vi "上管柱组件装配.vi"() -> ()   [LabVIEW 2020]
uses:
  Global_Variable/Global.vi
  Database/Global1.vi
  Global_Variable/A131258.vi
  <vilib>/addons/database/Connection.llb/DB Tools Open Connec (String).vi
  <vilib>/addons/database/Connection.llb/Conn Execute.vi
  <vilib>/addons/database/Recordset.llb/Rec Fetch Recordset Data (R).vi
  <vilib>/Utility/config.llb/NI_LVConfig.lvlib
  <vilib>/addons/database/NI_Database_API.lvlib
panel:
  out "USER_ID":string
  out "codeid":string
  out "deviceid":string
  out "productid":string
  out "产品型号":string
  out "联机模式":string
  out "用户权限":string
  out "用户名":string
  in  "轴承压装报表":string[][](table)=[["mm"], ["mm/s"]]
  in  "轴承压装判定结果":bool[][](array[boolean])=[[TRUE]]
  in  "选项卡控件 2":enum32{"轴承压装力位移曲线", "参数查看"}(tab)
  out "判定结果2 2":string
  out "判定结果1 2":string
  out "最小压力下限 2":dbl
  out "最小压力上限 2":dbl
  out "最大压力下限 2":dbl
  out "最大压力上限 2":dbl
  out "位移区间2内最小压力(KN)":dbl
  out "位移区间2内最大压力(KN)":dbl
  out "端铆判定结果45°":string
  out "端铆判定结果0°":string
  out "侧铆判定结果":string
  out "端铆最大压力45°上限":dbl
  out "端铆最大压力0°上限":dbl
  out "侧铆最大压力上限":dbl
  out "端铆最大压力45°下限":dbl
  out "端铆最大压力0°下限":dbl
  out "侧铆最大压力下限":dbl
  in  "质量报警":bool
  in  "设备缺料":bool
  in  "设备故障":bool
  out "端铆最大压力45°(KN)":dbl
  out "端铆最大压力0°(KN)":dbl
  out "侧铆最大压力(KN)":dbl
  out "判定结果3":string
  out "判定结果2":string
  out "判定结果1":string
  out "压装最终位移下限":dbl
  out "压装最终位移上限":dbl
  out "最小压力下限":dbl
  out "最小压力上限":dbl
  out "最大压力下限":dbl
  out "最大压力上限":dbl
  out "压装最终位移(mm)":dbl
  out "不合格指示灯":bool
  out "合格指示灯":bool
  out "位移区间1内最大压力(KN)":dbl
  out "位移区间1内最小压力(KN)":dbl
  out "产品条码":string
  out "轴承压装力位移曲线":cluster{dbl[], dbl[]}[](graph)
  in  "删除":bool
  in  "确定":bool
  in  "添加":bool
  in  "退出":bool
  in  "更新":bool
  in  "产品型号":string(combo)
  in  "选项卡控件 3":enum32{"轴承压装参数", "产品管理", "用户管理"}(tab)
  in  "坐标轴参数":string[][](table)=[["mm"], ["mm/s"]]
  in  "判定框参数":string[][](table)=[["mm"], ["mm/s"]]
  in  "结果判定参数":string[][](table)=[["mm"], ["mm/s"]]
  in  "请输入添加的产品名称":string
  in  "请选择要删除的产品":string(combo)
  in  "进入用户管理":bool
  # "上管柱组件装配"
  # "压装/铆接结果"
  # "下限值"
  # "上限值"
  # "判定结果"
  # "生产结果"
  # "产品二维码"
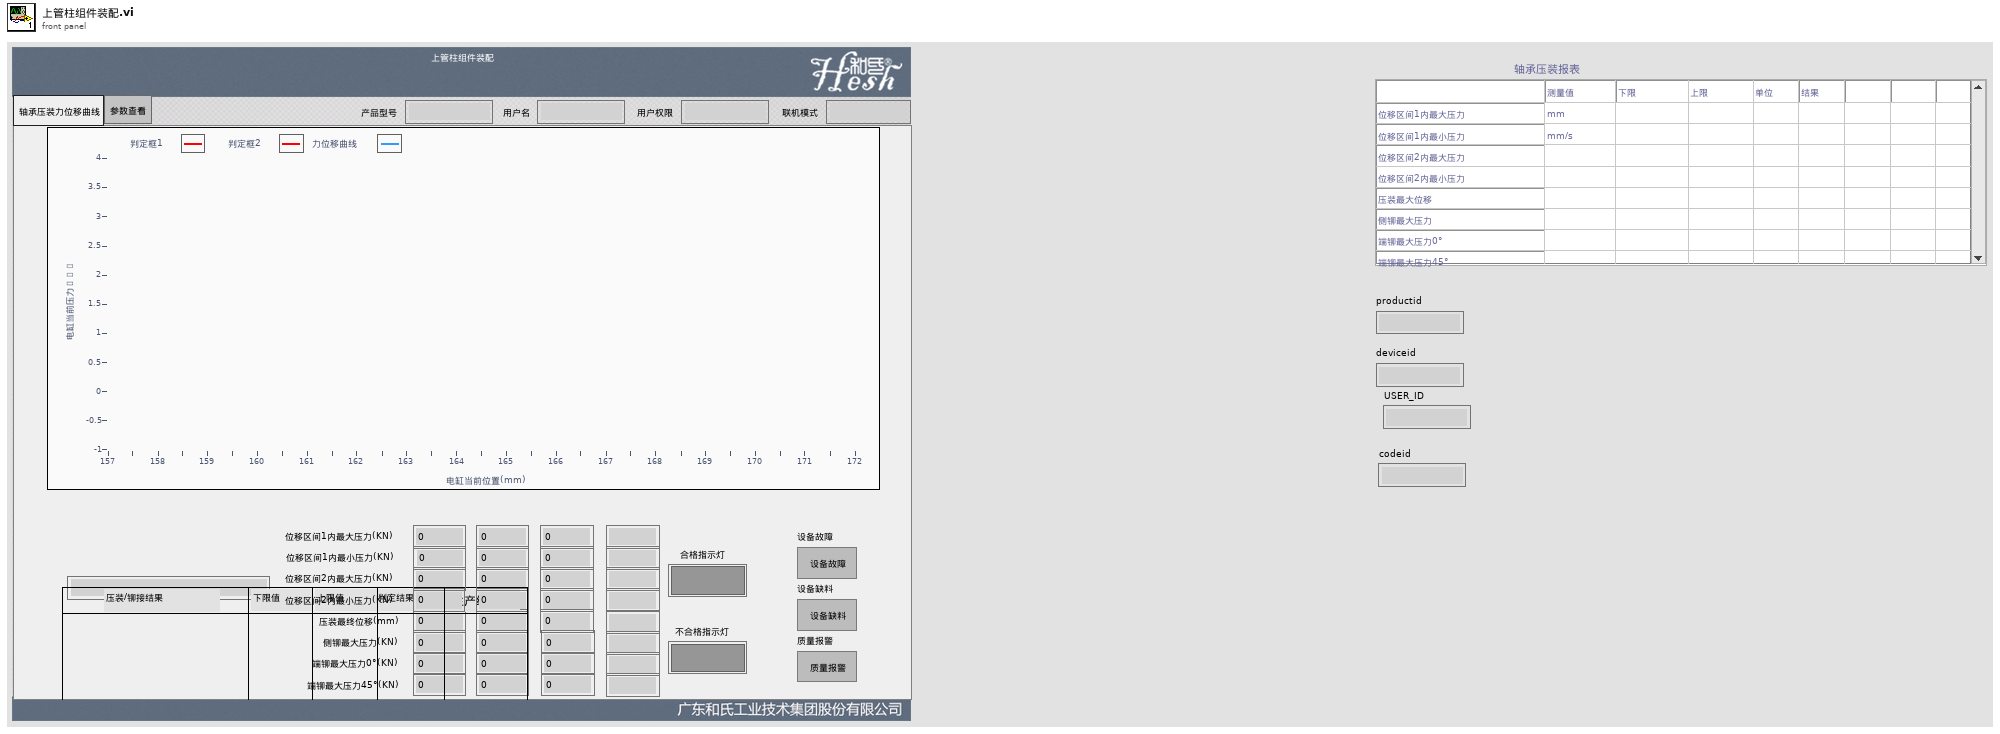
[diagram p1: front panel]
types:
  T1 = enum32{"Invalid", "Standard", "Closed", "Hidden", "Minimized", "Maximized"}
  T2 = cluster{"用户编号":string, "用户名":string, "用户密码(密文)":string, "用户权限":string}
  T3 = cluster{"设备名称":string, "用户名":string, "设备状态":enum16{"设备离线", "设备正常", "设备缺料", "设备故障", "质量报警"}, "附加信息":string}
  T4 = typedef "NI_LVConfig.lvlib/Config Data RefNum.ctl" = refnum<k1>
  T5 = typedef "NI_Database_API.lvlib/Conn ObjectReference.ctl" = refnum<k1>
  T6 = typedef "NI_Database_API.lvlib/Rec ObjectReference.ctl" = refnum<k1>
  T7 = cluster{i64, i64, i64, string, "result string":string}
  T8 = cluster{i64, i64, i64, string, "result string":string}[]
  T9 = cluster{i64, i64, string, "位移区间2内最小压力(KN)":dbl, "最小压力下限 2":dbl, "最小压力上限 2":dbl, string, "判定结果2 2":string}
  T10 = cluster{i64, i64, string, "位移区间2内最大压力(KN)":dbl, "最大压力下限 2":dbl, "最大压力上限 2":dbl, string, "判定结果1 2":string}
  T11 = cluster{i64, i64, string, "压装最终位移(mm) ":dbl, "压装最终位移下限":dbl, "压装最终位移上限":dbl, string, "判定结果3":string}
  T12 = cluster{i64, i64, string, "侧铆最大压力(KN)":dbl, "侧铆最大压力下限":dbl, "侧铆最大压力上限":dbl, string, "侧铆判定结果":string}
  T13 = cluster{i64, i64, string, "位移区间1内最小压力(KN)":dbl, "最小压力下限":dbl, "最小压力上限":dbl, string, "判定结果2":string}
  T14 = cluster{i64, i64, string, "端铆最大压力0°(KN)":dbl, "端铆最大压力0°下限":dbl, "端铆最大压力0°上限":dbl, string, "端铆判定结果0°":string}
  T15 = cluster{i64, i64, string, "位移区间1内最大压力(KN)":dbl, "最大压力下限":dbl, "最大压力上限":dbl, string, "判定结果1":string}
  T16 = cluster{i64, i64, string, "端铆最大压力45°(KN)":dbl, "端铆最大压力45°下限":dbl, "端铆最大压力45°上限":dbl, string, "端铆判定结果45°":string}
  T17 = cluster{i64, i64, string, "端铆最大压力45°(KN)":dbl, "端铆最大压力45°下限":dbl, "端铆最大压力45°上限":dbl, string, "端铆判定结果45°":string}[]
  T18 = cluster{i64, i64, "端铆最大压力45°(KN)":dbl, "端铆最大压力45°下限":dbl, "端铆最大压力45°上限":dbl, string, "端铆判定结果45°":string}
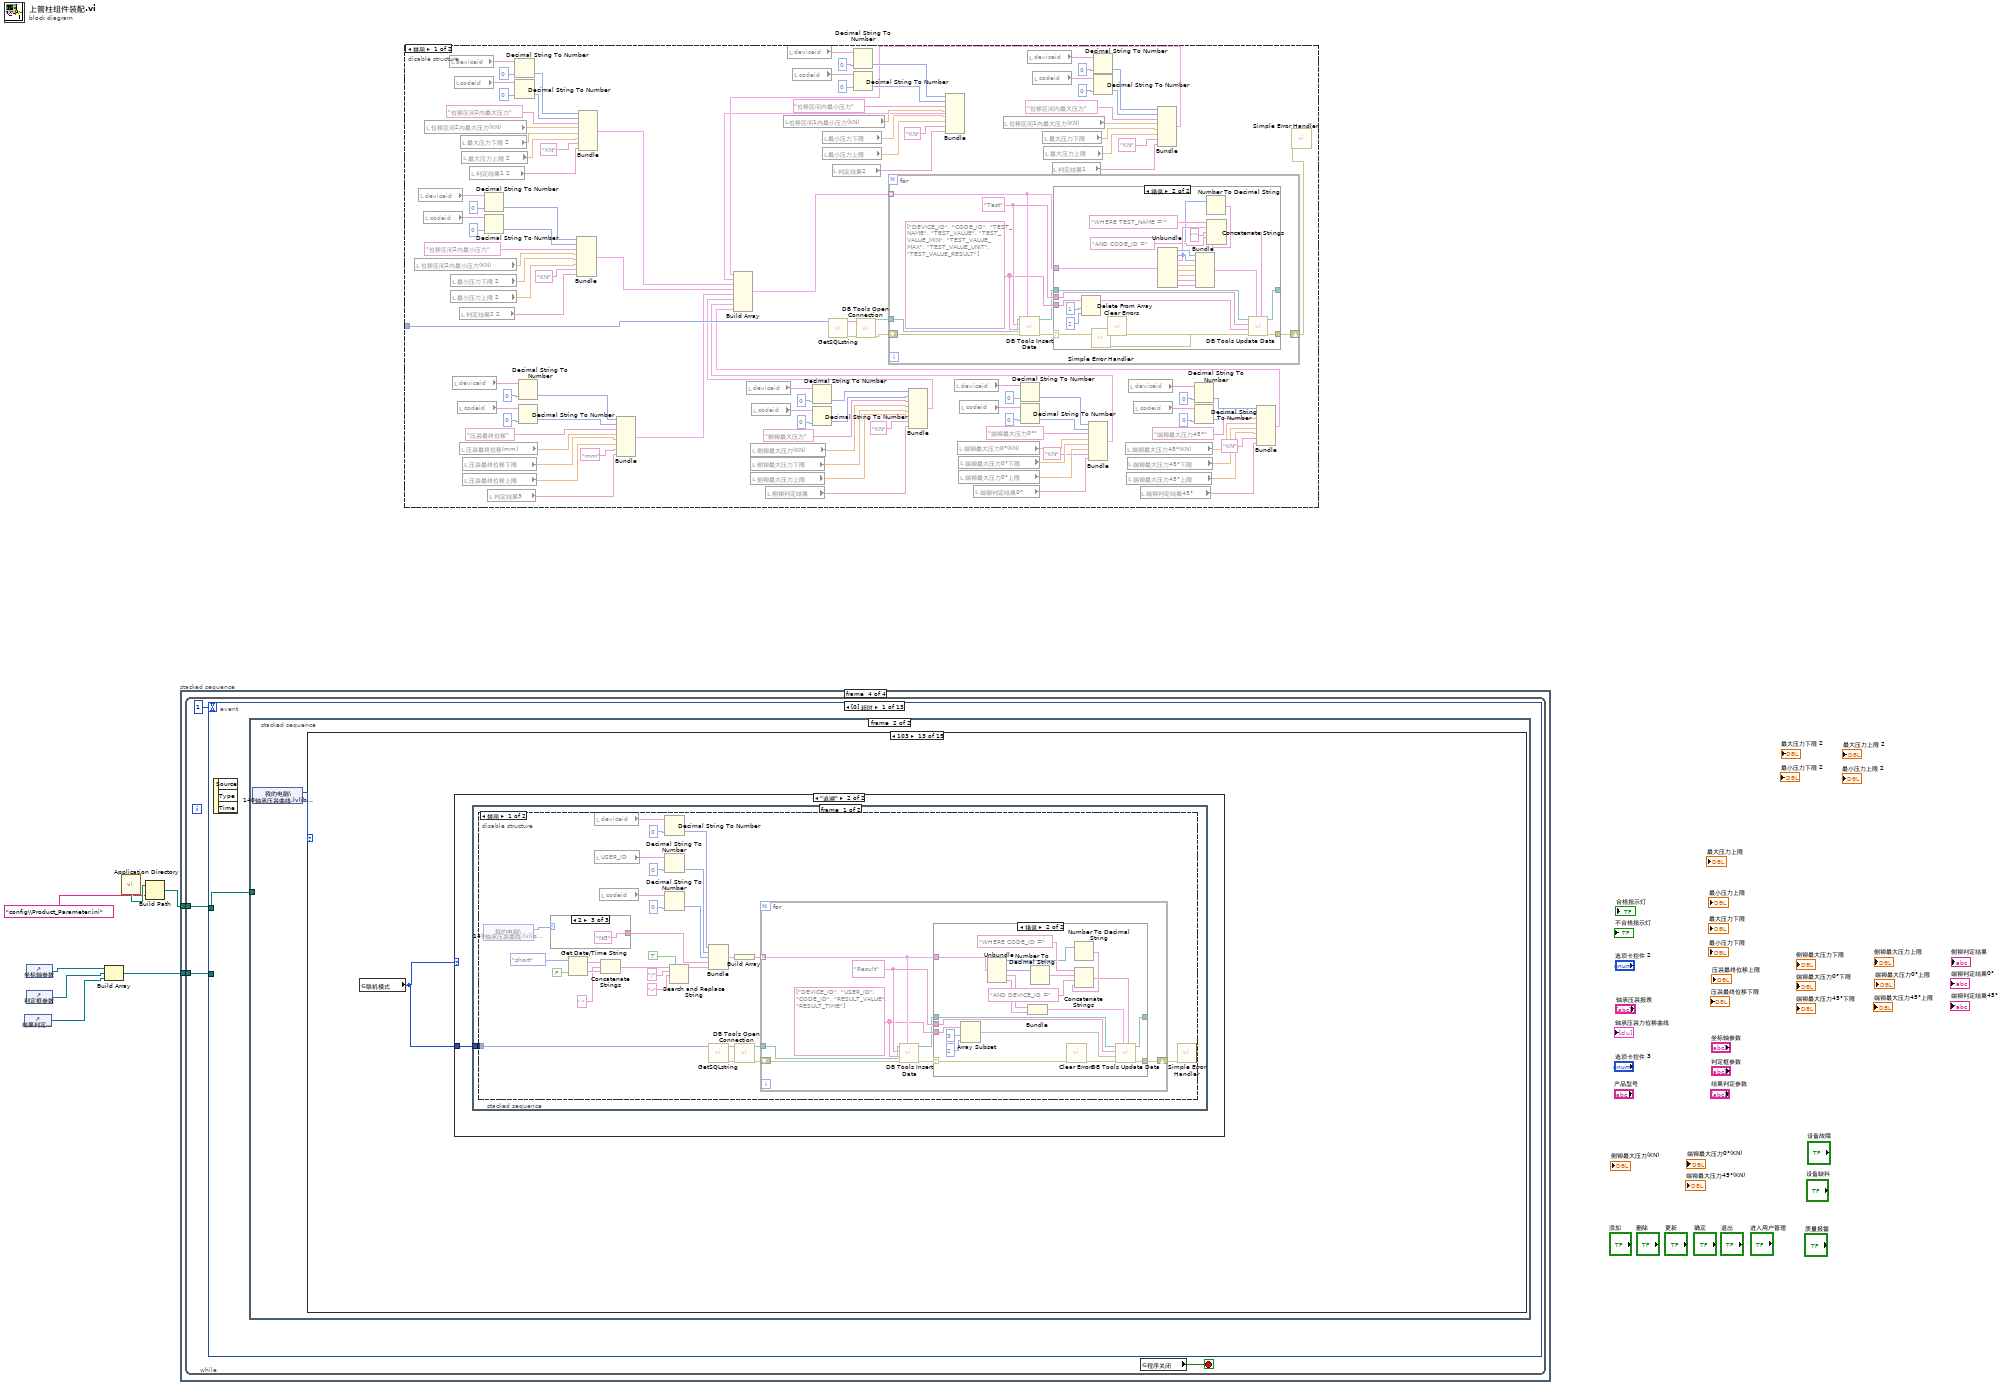
[diagram p0: block diagram]
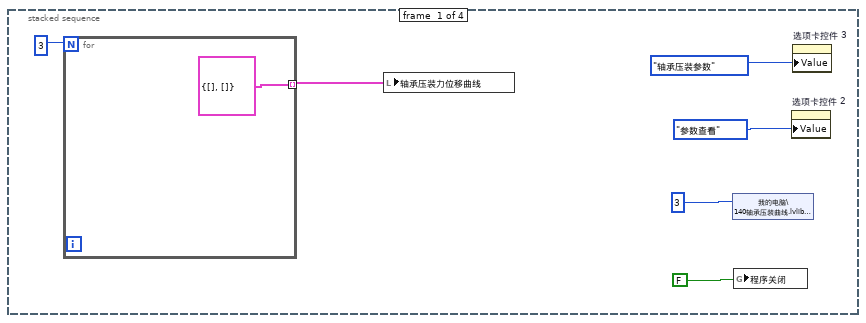
[diagram p4: hidden frame]
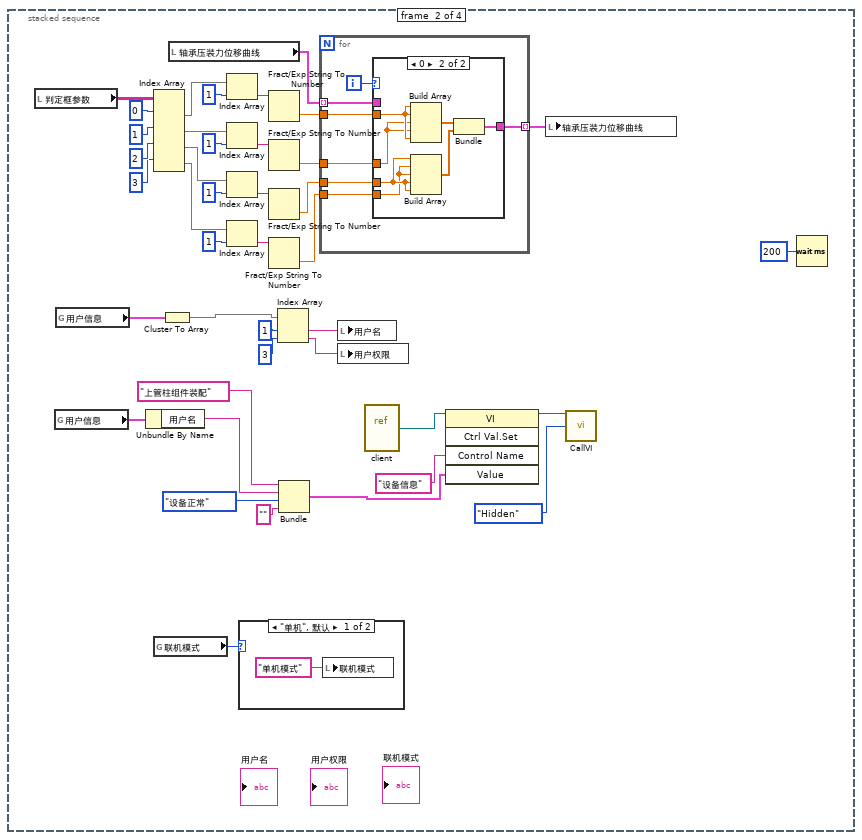
[diagram p5: hidden frame]
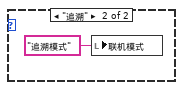
[diagram p6: hidden frame]
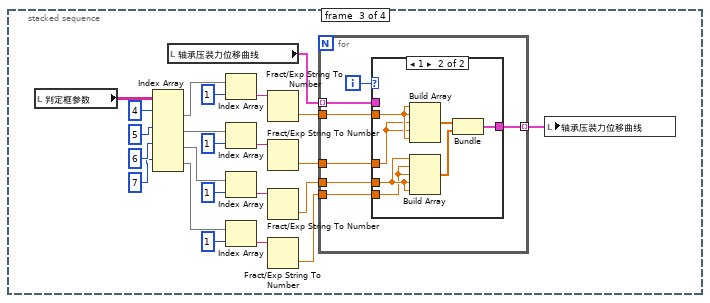
[diagram p8: hidden frame]
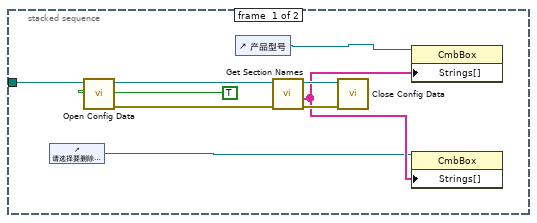
[diagram p10: hidden frame]
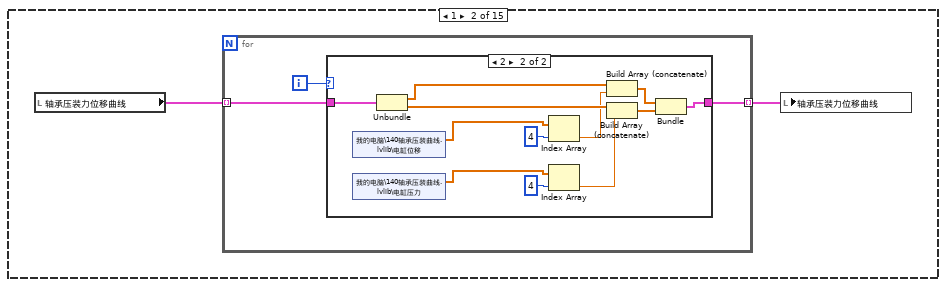
[diagram p12: hidden frame]
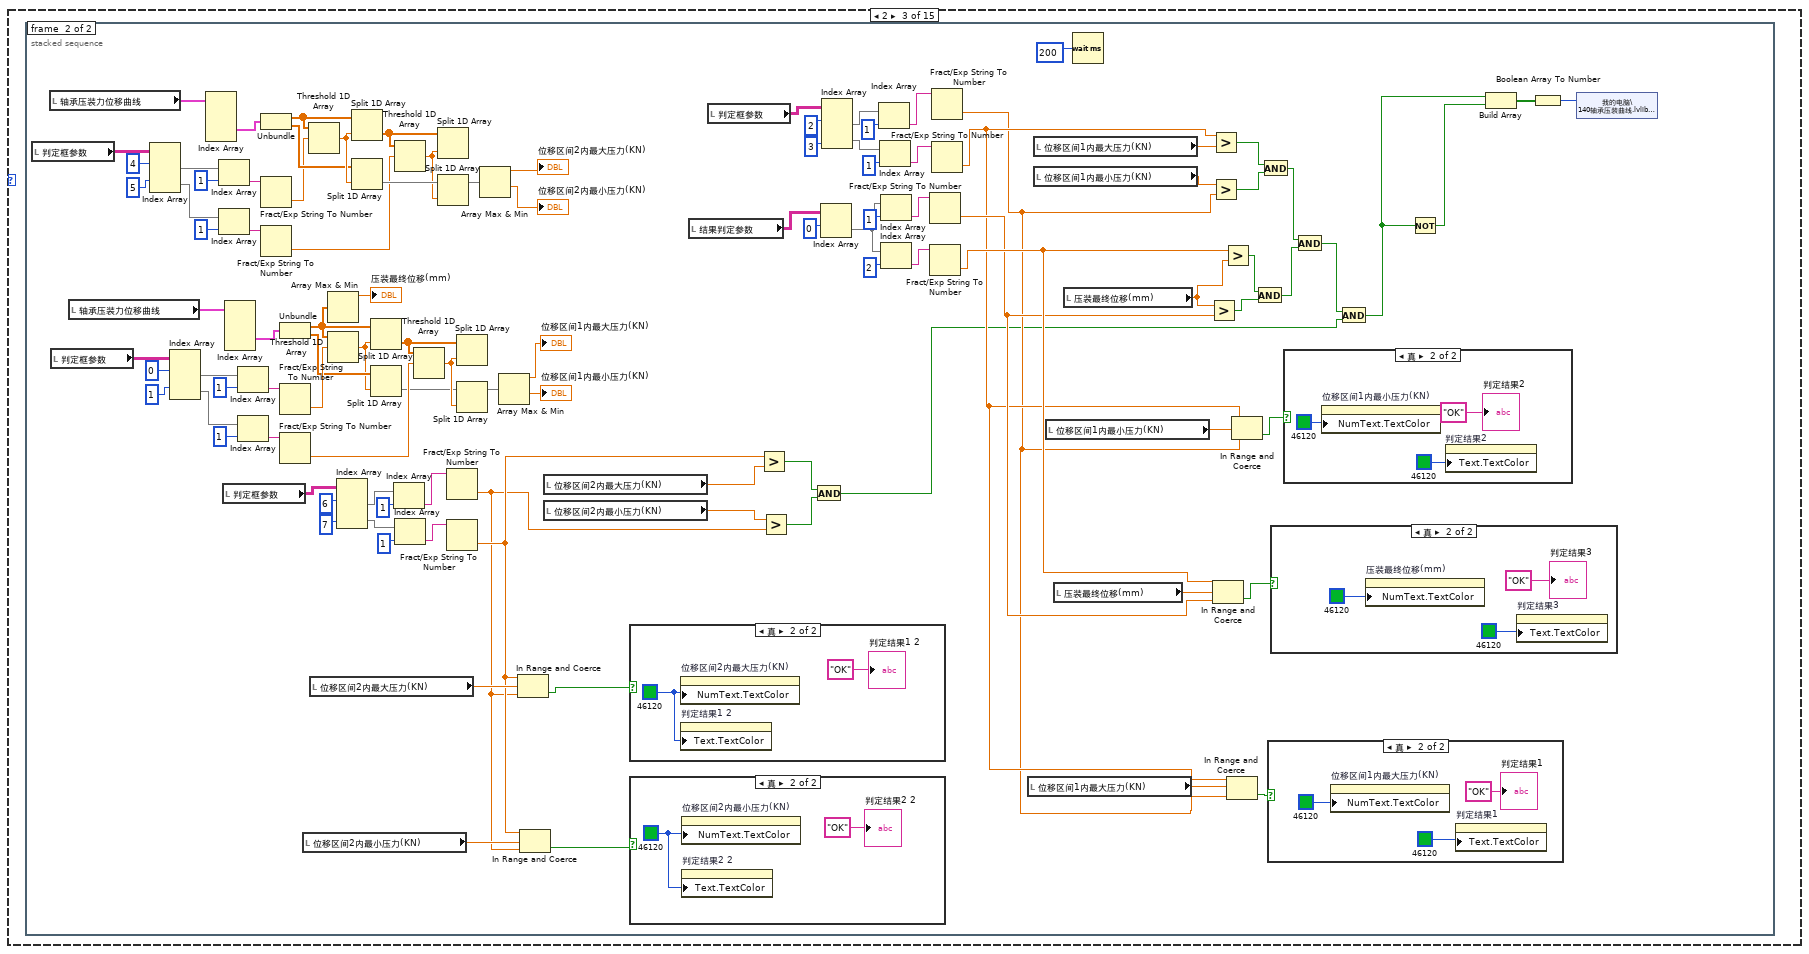
[diagram p14: hidden frame]
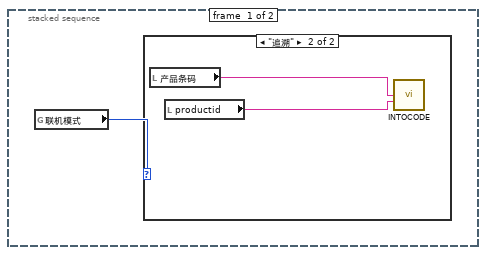
[diagram p15: hidden frame]
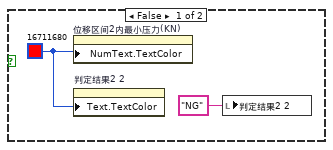
[diagram p17: hidden frame]
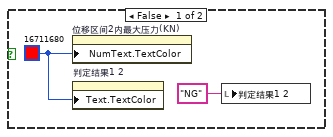
[diagram p18: hidden frame]
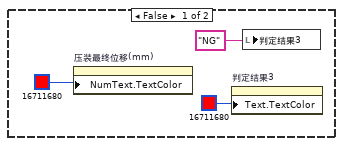
[diagram p19: hidden frame]
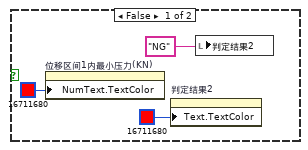
[diagram p20: hidden frame]
diagram:
  n1 = control-ref of="结果判定参数"() -> (w2:refnum<vi>)
  n2 = control-ref of="坐标轴参数"() -> (w4:refnum<vi>)
  n3 = control-ref of="判定框参数"() -> (w3:refnum<vi>)
  n4 = Build Array(w4, w3, w2) -> (w1:refnum<vi>[])
  n5 = call <vilib>:"Application Directory.vi"() -> ("Application Directory"=w7:path)
  n6 = Build Path(base path=w7, name or relative path="config\\Product_Parameter.ini" ("名称或相对路径")) -> (appended path=w5:path)
  n7 = stacked-sequence {
    tunnel: w5 -> [_ _ _ w112]
    tunnel: w1 -> [_ _ _ w111]
    frame #0 {
      n8 = for {
        N: 3 -> [_]
        tunnel: [cluster{dbl[], dbl[]} {[], []}] -> w11 mode=indexing
      }
      n9 = local write "轴承压装力位移曲线"(w11) -> ()
      n10 = shared-variable "我的电脑\\140轴承压装曲线.lvlib\\备用_1"(3) -> ()  [unwired: 1 in, 1 out]
      n11 = global write "Global.vi" "程序关闭"(FALSE ("程序关闭")) -> ()
      n12 = property on="选项卡控件 2" class="TabCtl (严格)"("Value"=enum32{"轴承压装力位移曲线", "参数查看"}."参数查看" ("选项卡控件 2")) -> ()  [unwired: 2 in, 2 out]
      n13 = property on="选项卡控件 3" class="TabCtl (严格)"("Value"=enum32{"轴承压装参数", "产品管理", "用户管理"}."轴承压装参数" ("选项卡控件 3")) -> ()  [unwired: 2 in, 2 out]
    }
    frame #1 {
      n14 = local read "判定框参数"() -> (w53:string[][])
      n15 = global read "Global1.vi" "用户信息"() -> (w23:T2)
      n16 = global read "Global1.vi" "用户信息"() -> (w32:T2)
      n17 = Unbundle By Name(w23) -> ("用户名"=w22:string)
      n18 = Index Array(array=w53, index (row) #1=0 ("索引 (行)"), index (row) #2=1 ("索引 (行)"), index (row) #3=2 ("索引 (行)"), index (row) #4=3 ("索引 (行)")) -> (element #1=w47:string[], element #2=w45:string[], element #3=w43:string[], element #4=w41:string[])  [unwired: 4 in]
      n19 = global read "Global1.vi" "联机模式"() -> (w26:enum16{"单机", "追溯"})
      n20 = Cluster To Array(cluster=w32) -> (array=w31:string[])
      n21 = local read "轴承压装力位移曲线"() -> (w55:cluster{dbl[], dbl[]}[])
      n22 = Index Array(array=w47, index=1 ("索引")) -> (element=w37:string)
      n23 = Index Array(array=w45, index=1 ("索引")) -> (element=w38:string)
      n24 = Index Array(array=w43, index=1 ("索引")) -> (element=w39:string)
      n25 = Index Array(array=w41, index=1 ("索引")) -> (element=w40:string)
      n26 = case shown="\"单机\", 默认" w26 {
        frame "单机", Default {
          n27 = local write "联机模式"("单机模式" ("联机模式")) -> ()
        }
        frame "追溯" {
          n28 = local write "联机模式"("追溯模式" ("联机模式")) -> ()
        }
      }
      n29 = Fract/Exp String To Number(string=w37) -> (number=w36:dbl)  [unwired: 3 in, 1 out]
      n30 = Fract/Exp String To Number(string=w38) -> (number=w35:dbl)  [unwired: 3 in, 1 out]
      n31 = Fract/Exp String To Number(string=w39) -> (number=w34:dbl)  [unwired: 3 in, 1 out]
      n32 = Fract/Exp String To Number(string=w40) -> (number=w33:dbl)  [unwired: 3 in, 1 out]
      n33 = Index Array(array=w31, index #1=1 ("索引"), index #2=3 ("索引")) -> (element #1=w28:string, element #2=w27:string)
      n34 = Bundle("设备名称"="上管柱组件装配", "用户名"=w22, "设备状态"=enum16{"设备离线", "设备正常", "设备缺料", "设备故障", "质量报警"}."设备正常", "附加信息"="") -> (w21:T3)  [unwired: 1 in]
      n35 = for {
        tunnel: [w64] -> w54 mode=indexing
        tunnel: w55 -> [w63] mode=indexing
        tunnel: w36 -> [w61]
        tunnel: w35 -> [w60]
        tunnel: w34 -> [w59]
        tunnel: w33 -> [w58]
        i -> [w62]
        n36 = case shown="0" w62 {
          tunnel: [w65 w70] -> w64
          tunnel: w63 -> [w65 _]
          tunnel: w61 -> [_ w69]
          tunnel: w60 -> [_ w68]
          tunnel: w59 -> [_ w67]
          tunnel: w58 -> [_ w66]
          frame Default {
          }
          frame 0 {
            n37 = Build Array(w69, w69, w68, w68, w69) -> (w71:dbl[])
            n38 = Build Array(w67, w66, w66, w67, w67) -> (w72:dbl[])
            n39 = Bundle(w71, w72) -> (w70:cluster{dbl[], dbl[]})  [unwired: 1 in]
          }
        }
      }
      n40 = local write "用户名"(w28) -> ()
      n41 = local write "用户权限"(w27) -> ()
      n42 = vi-ref "client.vi"() -> (w25:refnum<vi>)
      n43 = invoke class="VI" method="Ctrl Val.Set"(reference=w25, "Control Name"="设备信息" ("控件名"), "Value"=w21) -> (reference out=w24:refnum<vi>)  [unwired: 2 in, 4 out]
      n44 = local write "轴承压装力位移曲线"(w54) -> ()
      n45 = call "CallVI.vi"("VI引用"=w24, "状态"=T1."Hidden") -> ()  [unwired: 11 in, 3 out]
      n46 = Wait (ms)(milliseconds to wait=u32 200 ("等待时间（毫秒）")) -> ()  [unwired: 1 out]
    }
    frame #2 {
      n47 = local read "判定框参数"() -> (w83:string[][])
      n48 = Index Array(array=w83, index (row) #1=4 ("索引 (行)"), index (row) #2=5 ("索引 (行)"), index (row) #3=6 ("索引 (行)"), index (row) #4=7 ("索引 (行)")) -> (element #1=w84:string[], element #2=w85:string[], element #3=w86:string[], element #4=w87:string[])  [unwired: 4 in]
      n49 = local read "轴承压装力位移曲线"() -> (w81:cluster{dbl[], dbl[]}[])
      n50 = Index Array(array=w84, index=1 ("索引")) -> (element=w91:string)
      n51 = Index Array(array=w85, index=1 ("索引")) -> (element=w90:string)
      n52 = Index Array(array=w86, index=1 ("索引")) -> (element=w89:string)
      n53 = Index Array(array=w87, index=1 ("索引")) -> (element=w88:string)
      n54 = Fract/Exp String To Number(string=w91) -> (number=w92:dbl)  [unwired: 3 in, 1 out]
      n55 = Fract/Exp String To Number(string=w90) -> (number=w93:dbl)  [unwired: 3 in, 1 out]
      n56 = Fract/Exp String To Number(string=w89) -> (number=w94:dbl)  [unwired: 3 in, 1 out]
      n57 = Fract/Exp String To Number(string=w88) -> (number=w95:dbl)  [unwired: 3 in, 1 out]
      n58 = for {
        tunnel: [w102] -> w82 mode=indexing
        tunnel: w81 -> [w101] mode=indexing
        tunnel: w92 -> [w99]
        tunnel: w93 -> [w98]
        tunnel: w94 -> [w97]
        tunnel: w95 -> [w96]
        i -> [w100]
        n59 = case shown="1" w100 {
          tunnel: [w103 w108] -> w102
          tunnel: w101 -> [w103 _]
          tunnel: w99 -> [_ w107]
          tunnel: w98 -> [_ w106]
          tunnel: w97 -> [_ w105]
          tunnel: w96 -> [_ w104]
          frame Default {
          }
          frame 1 {
            n60 = Build Array(w107, w107, w106, w106, w107) -> (w109:dbl[])
            n61 = Build Array(w105, w104, w104, w105, w105) -> (w110:dbl[])
            n62 = Bundle(w109, w110) -> (w108:cluster{dbl[], dbl[]})  [unwired: 1 in]
          }
        }
      }
      n63 = local write "轴承压装力位移曲线"(w82) -> ()
    }
    frame #3 {
      n64 = while {
        tunnel: w112 -> [w115]
        tunnel: w111 -> [w116]
        stop <- w113 stop-if-true
        n65 = event shown="[0] 超时" {
          selector: _ -> [_ _ _ _ _ _ _ _ _ _ _ _ _]
          dyn-events: _ -> [_ _ _ _ _ _ _ _ _ _ _ _ _]
          timeout: 1 -> [_ _ _ _ _ _ _ _ _ _ _ _ _]
          tunnel: w115 -> [w117 w769 _ w979 w997 _ w1008 _ _ _ _ _ _]
          tunnel: w116 -> [_ _ _ w978 w996 _ w1007 _ _ _ _ _ _]
          event Timeout {
            n66 = event-data() -> ()  [unwired: 1 in, 3 out]
            n67 = stacked-sequence {
              tunnel: w117 -> [w120 _]
              frame #0 {
                n68 = control-ref of="请选择要删除的产品"() -> (w118:refnum<vi>)
                n69 = call <vilib>:"Open Config Data.vi"("create file if necessary (T)"=TRUE, "configuration file path"=w120) -> ("error out"=w123:errorcluster, "refnum"=w122:T4)  [unwired: 7 in, 1 out]
                n70 = control-ref of="产品型号"() -> (w119:refnum<vi>)
                n71 = call <vilib>:"Get Section Names.vi"("error in (no error)"=w123, "refnum"=w122) -> ("error out"=w125:errorcluster, "section names"=w121:string[], "refnum out"=w124:T4)  [unwired: 7 in]
                n72 = call <vilib>:"Close Config Data.vi"("error in (no error)"=w125, "refnum"=w124) -> ()  [unwired: 8 in, 2 out]
                n73 = property on="属性节点" class="CmbBox"(reference=w119, "Strings[]"=w121) -> ()  [unwired: 1 in, 2 out]
                n74 = property on="属性节点" class="CmbBox"(reference=w118, "Strings[]"=w121) -> ()  [unwired: 1 in, 2 out]
              }
              frame #1 {
                n75 = shared-variable "我的电脑\\140轴承压装曲线.lvlib\\备用_1"() -> (w127:u16)  [unwired: 1 in, 1 out]
                n76 = case shown="103" w127 {
                  frame 0, Default {
                  }
                  frame 1 {
                    n77 = local read "轴承压装力位移曲线"() -> (w128:cluster{dbl[], dbl[]}[])
                    n78 = for {
                      tunnel: [w132] -> w129 mode=indexing
                      tunnel: w128 -> [w131] mode=indexing
                      i -> [w130]
                      n79 = case shown="2" w130 {
                        tunnel: [w133 w139] -> w132
                        tunnel: w131 -> [w133 w138]
                        frame Default {
                        }
                        frame 2 {
                          n80 = shared-variable "我的电脑\\140轴承压装曲线.lvlib\\电缸位移"() -> (w134:sgl[])  [unwired: 1 in, 1 out]
                          n81 = shared-variable "我的电脑\\140轴承压装曲线.lvlib\\电缸压力"() -> (w135:sgl[])  [unwired: 1 in, 1 out]
                          n82 = Unbundle(w138) -> (w143:dbl[], w142:dbl[])
                          n83 = Index Array(array=w134, index=4) -> (element=w136:sgl)
                          n84 = Index Array(array=w135, index=4) -> (element=w137:sgl)
                          n85 = Build Array (concatenate)(w143, w136) -> (w141:dbl[])
                          n86 = Build Array (concatenate)(w142, w137) -> (w140:dbl[])
                          n87 = Bundle(w141, w140) -> (w139:cluster{dbl[], dbl[]})  [unwired: 1 in]
                        }
                      }
                    }
                    n88 = local write "轴承压装力位移曲线"(w129) -> ()
                  }
                  frame 2 {
                    n89 = stacked-sequence {
                      frame #0 {
                        n90 = global read "Global1.vi" "联机模式"() -> (w146:enum16{"单机", "追溯"})
                        n91 = case shown="\"追溯\"" w146 {
                          frame "单机", Default {
                          }
                          frame "追溯" {
                            n92 = local read "产品条码"() -> (w147:string)
                            n93 = local read "productid"() -> (w148:string)
                            n94 = call "INTOCODE.vi"("CODE_MAIN"=w147, "PRODUCT_ID"=w148) -> ()  [unwired: 13 in, 1 out]
                          }
                        }
                      }
                      frame #1 {
                        n95 = local read "判定框参数"() -> (w161:string[][])
                        n96 = local read "轴承压装力位移曲线"() -> (w169:cluster{dbl[], dbl[]}[])
                        n97 = local read "判定框参数"() -> (w187:string[][])
                        n98 = local read "轴承压装力位移曲线"() -> (w176:cluster{dbl[], dbl[]}[])
                        n99 = Index Array(array=w161, index (row) #1=4 ("索引 (行)"), index (row) #2=5 ("索引 (行)")) -> (element #1=w160:string[], element #2=w159:string[])  [unwired: 2 in]
                        n100 = Index Array(array=w187, index (row) #1=0 ("索引 (行)"), index (row) #2=1 ("索引 (行)")) -> (element #1=w188:string[], element #2=w189:string[])  [unwired: 2 in]
                        n101 = Index Array(array=w169) -> (element #3=w150:cluster{dbl[], dbl[]})  [unwired: 4 in, 3 out]
                        n102 = Index Array(array=w160, index=1 ("索引")) -> (element=w158:string)
                        n103 = Index Array(array=w159, index=1 ("索引")) -> (element=w157:string)
                        n104 = local read "判定框参数"() -> (w208:string[][])
                        n105 = Index Array(array=w176) -> (element #3=w149:cluster{dbl[], dbl[]})  [unwired: 4 in, 3 out]
                        n106 = Index Array(array=w188, index=1 ("索引")) -> (element=w190:string)
                        n107 = Index Array(array=w189, index=1 ("索引")) -> (element=w191:string)
                        n108 = Unbundle(w150) -> (w162:dbl[], w163:dbl[])
                        n109 = Fract/Exp String To Number(string=w158) -> (number=w156:dbl)  [unwired: 3 in, 1 out]
                        n110 = Fract/Exp String To Number(string=w157) -> (number=w155:dbl)  [unwired: 3 in, 1 out]
                        n111 = Unbundle(w149) -> (w185:dbl[], w184:dbl[])
                        n112 = Fract/Exp String To Number(string=w190) -> (number=w192:dbl)  [unwired: 3 in, 1 out]
                        n113 = Fract/Exp String To Number(string=w191) -> (number=w193:dbl)  [unwired: 3 in, 1 out]
                        n114 = local read "位移区间2内最小压力(KN)"() -> (w198:dbl)
                        n115 = Threshold 1D Array(2:w156, 3:w162) -> (0:w168:dbl)  [unwired: 1 in]
                        n116 = local read "位移区间2内最大压力(KN)"() -> (w200:dbl)
                        n117 = Array Max & Min(array=w185) -> (max value=→"压装最终位移(mm)":dbl)  [unwired: 3 out]
                        n118 = Threshold 1D Array(2:w192, 3:w185) -> (0:w177:dbl)  [unwired: 1 in]
                        n119 = Index Array(array=w208, index (row) #1=6 ("索引 (行)"), index (row) #2=7 ("索引 (行)")) -> (element #1=w211:string[], element #2=w213:string[])  [unwired: 2 in]
                        n120 = Split 1D Array(array=w162, index=w168) -> (second subarray=w166:dbl[])  [unwired: 1 out]
                        n121 = Split 1D Array(array=w163, index=w168) -> (second subarray=w167:dbl[])  [unwired: 1 out]
                        n122 = Split 1D Array(array=w185, index=w177) -> (second subarray=w179:dbl[])  [unwired: 1 out]
                        n123 = Split 1D Array(array=w184, index=w177) -> (second subarray=w178:dbl[])  [unwired: 1 out]
                        n124 = Index Array(array=w211, index=1 ("索引")) -> (element=w215:string)
                        n125 = Threshold 1D Array(2:w155, 3:w166) -> (0:w165:dbl)  [unwired: 1 in]
                        n126 = Index Array(array=w213, index=1 ("索引")) -> (element=w216:string)
                        n127 = Threshold 1D Array(2:w193, 3:w179) -> (0:w180:dbl)  [unwired: 1 in]
                        n128 = Split 1D Array(array=w166, index=w165) -> ()  [unwired: 2 out]
                        n129 = Split 1D Array(array=w167, index=w165) -> (first subarray=w164:dbl[])  [unwired: 1 out]
                        n130 = Fract/Exp String To Number(string=w215) -> (number=w195:dbl)  [unwired: 3 in, 1 out]
                        n131 = Fract/Exp String To Number(string=w216) -> (number=w196:dbl)  [unwired: 3 in, 1 out]
                        n132 = Split 1D Array(array=w179, index=w180) -> ()  [unwired: 2 out]
                        n133 = Split 1D Array(array=w178, index=w180) -> (first subarray=w181:dbl[])  [unwired: 1 out]
                        n134 = Array Max & Min(array=w164) -> (max value=→"位移区间2内最大压力(KN)":dbl, min value=→"位移区间2内最小压力(KN)":dbl)  [unwired: 2 out]
                        n135 = Array Max & Min(array=w181) -> (max value=→"位移区间1内最大压力(KN)":dbl, min value=→"位移区间1内最小压力(KN)":dbl)  [unwired: 2 out]
                        n136 = In Range and Coerce(upper limit=w196, x=w200, lower limit=w195) -> (In Range?=w199:bool)  [unwired: 1 out]
                        n137 = In Range and Coerce(upper limit=w196, x=w198, lower limit=w195) -> (In Range?=w197:bool)  [unwired: 1 out]
                        n138 = local read "位移区间2内最大压力(KN)"() -> (w207:dbl)
                        n139 = local read "位移区间2内最小压力(KN)"() -> (w206:dbl)
                        n140 = case shown="真" w199 {
                          frame False {
                            w259 = u32 16711680
                            n141 = property on="位移区间2内最大压力(KN)" class="DigNum (严格)"("NumText.TextColor"=w259) -> ()  [unwired: 2 in, 2 out]
                            n142 = property on="判定结果1 2" class="Str"("Text.TextColor"=w259) -> ()  [unwired: 2 in, 2 out]
                            n143 = local write "判定结果1 2"("NG" ("判定结果1")) -> ()
                          }
                          frame True {
                            w261 = u32 46120
                            n144 = property on="位移区间2内最大压力(KN)" class="DigNum (严格)"("NumText.TextColor"=w261) -> ()  [unwired: 2 in, 2 out]
                            n145 = property on="判定结果1 2" class="Str"("Text.TextColor"=w261) -> ()  [unwired: 2 in, 2 out]
                            "判定结果1 2" <- "OK" ("判定结果1")
                          }
                        }
                        n146 = case shown="真" w197 {
                          frame False {
                            w255 = u32 16711680
                            n147 = property on="位移区间2内最小压力(KN)" class="DigNum (严格)"("NumText.TextColor"=w255) -> ()  [unwired: 2 in, 2 out]
                            n148 = property on="判定结果2 2" class="Str"("Text.TextColor"=w255) -> ()  [unwired: 2 in, 2 out]
                            n149 = local write "判定结果2 2"("NG" ("判定结果1")) -> ()
                          }
                          frame True {
                            w257 = u32 46120
                            n150 = property on="位移区间2内最小压力(KN)" class="DigNum (严格)"("NumText.TextColor"=w257) -> ()  [unwired: 2 in, 2 out]
                            n151 = property on="判定结果2 2" class="Str"("Text.TextColor"=w257) -> ()  [unwired: 2 in, 2 out]
                            "判定结果2 2" <- "OK" ("判定结果1")
                          }
                        }
                        n152 = local read "结果判定参数"() -> (w227:string[][])
                        n153 = local read "判定框参数"() -> (w236:string[][])
                        n154 = Greater?(x=w196, y=w207) -> (0:w205:bool)
                        n155 = Greater?(x=w206, y=w195) -> (0:w204:bool)
                        n156 = And(x=w205, y=w204) -> (x .and. y?=w202:bool)
                        n157 = Index Array(array=w227, index (row)=0 ("索引 (行)")) -> (element=w223:string[])  [unwired: 1 in]
                        n158 = Index Array(array=w236, index (row) #1=2 ("索引 (行)"), index (row) #2=3 ("索引 (行)")) -> (element #1=w233:string[], element #2=w231:string[])  [unwired: 2 in]
                        n159 = Index Array(array=w233, index=1 ("索引")) -> (element=w229:string)
                        n160 = Index Array(array=w231, index=1 ("索引")) -> (element=w228:string)
                        n161 = Index Array(array=w223, index=1 ("索引")) -> (element=w224:string)
                        n162 = Index Array(array=w223, index=2 ("索引")) -> (element=w221:string)
                        n163 = Fract/Exp String To Number(string=w224) -> (number=w219:dbl)  [unwired: 3 in, 1 out]
                        n164 = Fract/Exp String To Number(string=w221) -> (number=w220:dbl)  [unwired: 3 in, 1 out]
                        n165 = Fract/Exp String To Number(string=w229) -> (number=w217:dbl)  [unwired: 3 in, 1 out]
                        n166 = Fract/Exp String To Number(string=w228) -> (number=w218:dbl)  [unwired: 3 in, 1 out]
                        n167 = local read "位移区间1内最大压力(KN)"() -> (w242:dbl)
                        n168 = local read "位移区间1内最大压力(KN)"() -> (w251:dbl)
                        n169 = local read "位移区间1内最小压力(KN)"() -> (w250:dbl)
                        n170 = local read "位移区间1内最小压力(KN)"() -> (w240:dbl)
                        n171 = local read "压装最终位移(mm)"() -> (w238:dbl)
                        n172 = local read "压装最终位移(mm)"() -> (w243:dbl)
                        n173 = Wait (ms)(milliseconds to wait=u32 200 ("等待时间（毫秒）")) -> ()  [unwired: 1 out]
                        n174 = Greater?(x=w243, y=w219) -> (0:w247:bool)
                        n175 = Greater?(x=w218, y=w251) -> (0:w249:bool)
                        n176 = Greater?(x=w250, y=w217) -> (0:w248:bool)
                        n177 = In Range and Coerce(upper limit=w220, x=w238, lower limit=w219) -> (In Range?=w237:bool)  [unwired: 1 out]
                        n178 = Greater?(x=w220, y=w243) -> (0:w244:bool)
                        n179 = In Range and Coerce(upper limit=w218, x=w242, lower limit=w217) -> (In Range?=w241:bool)  [unwired: 1 out]
                        n180 = In Range and Coerce(upper limit=w218, x=w240, lower limit=w217) -> (In Range?=w239:bool)  [unwired: 1 out]
                        n181 = And(x=w244, y=w247) -> (x .and. y?=w245:bool)
                        n182 = And(x=w249, y=w248) -> (x .and. y?=w246:bool)
                        n183 = case shown="真" w241 {
                          frame False {
                            n184 = property on="位移区间1内最大压力(KN)" class="DigNum (严格)"("NumText.TextColor"=u32 16711680) -> ()  [unwired: 2 in, 2 out]
                            n185 = property on="判定结果1" class="Str"("Text.TextColor"=u32 16711680) -> ()  [unwired: 2 in, 2 out]
                            n186 = local write "判定结果1"("NG" ("判定结果1")) -> ()
                          }
                          frame True {
                            n187 = property on="位移区间1内最大压力(KN)" class="DigNum (严格)"("NumText.TextColor"=u32 46120) -> ()  [unwired: 2 in, 2 out]
                            n188 = property on="判定结果1" class="Str"("Text.TextColor"=u32 46120) -> ()  [unwired: 2 in, 2 out]
                            "判定结果1" <- "OK" ("判定结果1")
                          }
                        }
                        n189 = case shown="真" w237 {
                          frame False {
                            n190 = property on="压装最终位移(mm)" class="DigNum (严格)"("NumText.TextColor"=u32 16711680) -> ()  [unwired: 2 in, 2 out]
                            n191 = property on="判定结果3" class="Str"("Text.TextColor"=u32 16711680) -> ()  [unwired: 2 in, 2 out]
                            n192 = local write "判定结果3"("NG" ("判定结果1")) -> ()
                          }
                          frame True {
                            n193 = property on="压装最终位移(mm)" class="DigNum (严格)"("NumText.TextColor"=u32 46120) -> ()  [unwired: 2 in, 2 out]
                            n194 = property on="判定结果3" class="Str"("Text.TextColor"=u32 46120) -> ()  [unwired: 2 in, 2 out]
                            "判定结果3" <- "OK" ("判定结果1")
                          }
                        }
                        n195 = case shown="真" w239 {
                          frame False {
                            n196 = property on="位移区间1内最小压力(KN)" class="DigNum (严格)"("NumText.TextColor"=u32 16711680) -> ()  [unwired: 2 in, 2 out]
                            n197 = property on="判定结果2" class="Str"("Text.TextColor"=u32 16711680) -> ()  [unwired: 2 in, 2 out]
                            n198 = local write "判定结果2"("NG" ("判定结果1")) -> ()
                          }
                          frame True {
                            n199 = property on="位移区间1内最小压力(KN)" class="DigNum (严格)"("NumText.TextColor"=u32 46120) -> ()  [unwired: 2 in, 2 out]
                            n200 = property on="判定结果2" class="Str"("Text.TextColor"=u32 46120) -> ()  [unwired: 2 in, 2 out]
                            "判定结果2" <- "OK" ("判定结果1")
                          }
                        }
                        n201 = And(x=w246, y=w245) -> (x .and. y?=w203:bool)
                        n202 = And(x=w203, y=w202) -> (x .and. y?=w201:bool)
                        n203 = Not(x=w201) -> (.not. x?=w252:bool)
                        n204 = Build Array(w201, w252) -> (w254:bool[])
                        n205 = Boolean Array To Number(Boolean array=w254) -> (number=w253:u32)
                        n206 = shared-variable "我的电脑\\140轴承压装曲线.lvlib\\备用_2"(w253) -> ()  [unwired: 1 in, 1 out]
                      }
                    }
                  }
                  frame 3 {
                    w284 = u32 0
                    w282 = "" ("判定结果2")
                    w296 = u16 0 ("备用_2")
                    w349 = FALSE
                    w283 = nan
                    n207 = local read "判定框参数"() -> (w348:string[][])
                    n208 = local read "判定框参数"() -> (w285:string[][])
                    n209 = shared-variable "我的电脑\\140轴承压装曲线.lvlib\\备用_3"(w296) -> ()  [unwired: 1 in, 1 out]
                    n210 = shared-variable "我的电脑\\140轴承压装曲线.lvlib\\备用_4"(w296) -> ()  [unwired: 1 in, 1 out]
                    n211 = shared-variable "我的电脑\\140轴承压装曲线.lvlib\\备用_5"(w296) -> ()  [unwired: 1 in, 1 out]
                    n212 = shared-variable "我的电脑\\140轴承压装曲线.lvlib\\备用_6"(w296) -> ()  [unwired: 1 in, 1 out]
                    n213 = shared-variable "我的电脑\\140轴承压装曲线.lvlib\\备用_7"(w296) -> ()  [unwired: 1 in, 1 out]
                    n214 = Index Array(array=w348, index (row) #1=2 ("索引 (行)"), index (row) #2=3 ("索引 (行)")) -> (element #1=w345:string[], element #2=w343:string[])  [unwired: 2 in]
                    n215 = Index Array(array=w285, index (row) #1=6 ("索引 (行)"), index (row) #2=7 ("索引 (行)")) -> (element #1=w288:string[], element #2=w290:string[])  [unwired: 2 in]
                    n216 = Index Array(array=w345, index=1 ("索引")) -> (element=w341:string)
                    n217 = Index Array(array=w343, index=1 ("索引")) -> (element=w340:string)
                    n218 = Index Array(array=w288, index=1 ("索引")) -> (element=w292:string)
                    n219 = Index Array(array=w290, index=1 ("索引")) -> (element=w293:string)
                    n220 = Fract/Exp String To Number(string=w341) -> (number=w338:dbl)  [unwired: 3 in, 1 out]
                    n221 = Fract/Exp String To Number(string=w340) -> (number=w339:dbl)  [unwired: 3 in, 1 out]
                    n222 = Fract/Exp String To Number(string=w292) -> (number=w295:dbl)  [unwired: 3 in, 1 out]
                    n223 = Fract/Exp String To Number(string=w293) -> (number=w294:dbl)  [unwired: 3 in, 1 out]
                    n224 = local write "最大压力下限"(w338) -> ()
                    n225 = local write "最小压力下限"(w338) -> ()
                    n226 = local write "最大压力上限"(w339) -> ()
                    n227 = local write "最小压力上限"(w339) -> ()
                    n228 = local write "最大压力下限 2"(w295) -> ()
                    n229 = local write "最小压力下限 2"(w295) -> ()
                    n230 = local write "最大压力上限 2"(w294) -> ()
                    n231 = local write "最小压力上限 2"(w294) -> ()
                    n232 = for {
                      N: 3 -> [_]
                      tunnel: [cluster{dbl[], dbl[]} {[], []}] -> w352 mode=indexing
                    }
                    n233 = local read "结果判定参数"() -> (w333:string[][])
                    n234 = Index Array(array=w333, index (row) #1=0 ("索引 (行)"), index (row) #2=0 ("索引 (行)"), index (row) #3=1 ("索引 (行)"), index (row) #4=1 ("索引 (行)"), index (row) #5=2 ("索引 (行)"), index (row) #6=2 ("索引 (行)"), index (row) #7=3 ("索引 (行)"), index (row) #8=3 ("索引 (行)")) -> (element #1=w337:string[], element #2=w336:string[], element #3=w330:string[], element #4=w329:string[], element #5=w328:string[], element #6=w327:string[], element #7=w326:string[], element #8=w325:string[])  [unwired: 8 in]
                    n235 = local write "轴承压装力位移曲线"(w352) -> ()
                    n236 = shared-variable "我的电脑\\140轴承压装曲线.lvlib\\备用_1"(4) -> ()  [unwired: 1 in, 1 out]
                    n237 = Index Array(array=w337, index=1 ("索引")) -> (element=w335:string)
                    n238 = Index Array(array=w336, index=2 ("索引")) -> (element=w334:string)
                    n239 = Index Array(array=w330, index=1 ("索引")) -> (element=w324:string)
                    n240 = Index Array(array=w329, index=2 ("索引")) -> (element=w323:string)
                    n241 = Index Array(array=w328, index=1 ("索引")) -> (element=w322:string)
                    n242 = Index Array(array=w327, index=2 ("索引")) -> (element=w321:string)
                    n243 = Index Array(array=w326, index=1 ("索引")) -> (element=w320:string)
                    n244 = Index Array(array=w325, index=2 ("索引")) -> (element=w319:string)
                    n245 = local write "不合格指示灯"(w349) -> ()
                    n246 = local write "轴承压装判定结果"(bool[][] [] ("轴承压装判定结果")) -> ()
                    n247 = local write "合格指示灯"(w349) -> ()
                    n248 = Fract/Exp String To Number(string=w335) -> (number=w331:dbl)  [unwired: 3 in, 1 out]
                    n249 = Fract/Exp String To Number(string=w334) -> (number=w332:dbl)  [unwired: 3 in, 1 out]
                    n250 = Fract/Exp String To Number(string=w324) -> (number=w318:dbl)  [unwired: 3 in, 1 out]
                    n251 = Fract/Exp String To Number(string=w323) -> (number=w317:dbl)  [unwired: 3 in, 1 out]
                    n252 = Fract/Exp String To Number(string=w322) -> (number=w316:dbl)  [unwired: 3 in, 1 out]
                    n253 = Fract/Exp String To Number(string=w321) -> (number=w315:dbl)  [unwired: 3 in, 1 out]
                    n254 = Fract/Exp String To Number(string=w320) -> (number=w314:dbl)  [unwired: 3 in, 1 out]
                    n255 = Fract/Exp String To Number(string=w319) -> (number=w313:dbl)  [unwired: 3 in, 1 out]
                    n256 = local write "压装最终位移下限"(w331) -> ()
                    n257 = local write "压装最终位移上限"(w332) -> ()
                    n258 = local write "侧铆最大压力下限"(w318) -> ()
                    n259 = local write "侧铆最大压力上限"(w317) -> ()
                    n260 = local write "端铆最大压力0°下限"(w316) -> ()
                    n261 = local write "端铆最大压力0°上限"(w315) -> ()
                    n262 = local write "端铆最大压力45°下限"(w314) -> ()
                    n263 = local write "端铆最大压力45°上限"(w313) -> ()
                    n264 = local write "位移区间1内最大压力(KN)"(w283) -> ()
                    n265 = local write "位移区间1内最小压力(KN)"(w283) -> ()
                    n266 = local write "位移区间2内最大压力(KN)"(w283) -> ()
                    n267 = local write "位移区间2内最小压力(KN)"(w283) -> ()
                    n268 = local write "端铆最大压力45°(KN)"(w283) -> ()
                    n269 = local write "压装最终位移(mm)"(w283) -> ()
                    n270 = local write "侧铆最大压力(KN)"(w283) -> ()
                    n271 = local write "端铆最大压力0°(KN)"(w283) -> ()
                    n272 = property on="位移区间1内最大压力(KN)" class="DigNum (严格)"("NumText.TextColor"=w284) -> ()  [unwired: 2 in, 2 out]
                    n273 = property on="位移区间1内最小压力(KN)" class="DigNum (严格)"("NumText.TextColor"=w284) -> ()  [unwired: 2 in, 2 out]
                    n274 = property on="压装最终位移(mm)" class="DigNum (严格)"("NumText.TextColor"=w284) -> ()  [unwired: 2 in, 2 out]
                    n275 = property on="侧铆最大压力(KN)" class="DigNum (严格)"("NumText.TextColor"=w284) -> ()  [unwired: 2 in, 2 out]
                    n276 = property on="端铆最大压力0°(KN)" class="DigNum (严格)"("NumText.TextColor"=w284) -> ()  [unwired: 2 in, 2 out]
                    n277 = property on="端铆最大压力45°(KN)" class="DigNum (严格)"("NumText.TextColor"=w284) -> ()  [unwired: 2 in, 2 out]
                    n278 = property on="位移区间2内最大压力(KN)" class="DigNum (严格)"("NumText.TextColor"=w284) -> ()  [unwired: 2 in, 2 out]
                    n279 = property on="位移区间2内最小压力(KN)" class="DigNum (严格)"("NumText.TextColor"=w284) -> ()  [unwired: 2 in, 2 out]
                    n280 = local write "判定结果1"(w282) -> ()
                    n281 = local write "判定结果2"(w282) -> ()
                    n282 = local write "判定结果3"(w282) -> ()
                    n283 = local write "侧铆判定结果"(w282) -> ()
                    n284 = local write "端铆判定结果0°"(w282) -> ()
                    n285 = local write "端铆判定结果45°"(w282) -> ()
                    n286 = local write "判定结果1 2"(w282) -> ()
                    n287 = local write "判定结果2 2"(w282) -> ()
                  }
                  frame 4 {
                    n288 = stacked-sequence {
                      frame #0 {
                        n289 = local read "判定框参数"() -> (w358:string[][])
                        n290 = Index Array(array=w358, index (row) #1=0 ("索引 (行)"), index (row) #2=1 ("索引 (行)"), index (row) #3=2 ("索引 (行)"), index (row) #4=3 ("索引 (行)")) -> (element #1=w369:string[], element #2=w367:string[], element #3=w365:string[], element #4=w363:string[])  [unwired: 4 in]
                        n291 = local read "轴承压装力位移曲线"() -> (w375:cluster{dbl[], dbl[]}[])
                        n292 = Index Array(array=w369, index=1 ("索引")) -> (element=w359:string)
                        n293 = Index Array(array=w367, index=1 ("索引")) -> (element=w360:string)
                        n294 = Index Array(array=w365, index=1 ("索引")) -> (element=w361:string)
                        n295 = Index Array(array=w363, index=1 ("索引")) -> (element=w362:string)
                        n296 = Fract/Exp String To Number(string=w359) -> (number=w357:dbl)  [unwired: 3 in, 1 out]
                        n297 = Fract/Exp String To Number(string=w360) -> (number=w356:dbl)  [unwired: 3 in, 1 out]
                        n298 = Fract/Exp String To Number(string=w361) -> (number=w355:dbl)  [unwired: 3 in, 1 out]
                        n299 = Fract/Exp String To Number(string=w362) -> (number=w354:dbl)  [unwired: 3 in, 1 out]
                        n300 = for {
                          tunnel: [w383] -> w376 mode=indexing
                          tunnel: w375 -> [w382] mode=indexing
                          tunnel: w357 -> [w380]
                          tunnel: w356 -> [w379]
                          tunnel: w355 -> [w378]
                          tunnel: w354 -> [w377]
                          i -> [w381]
                          n301 = case shown="0" w381 {
                            tunnel: [w384 w389] -> w383
                            tunnel: w382 -> [w384 _]
                            tunnel: w380 -> [_ w388]
                            tunnel: w379 -> [_ w387]
                            tunnel: w378 -> [_ w386]
                            tunnel: w377 -> [_ w385]
                            frame Default {
                            }
                            frame 0 {
                              n302 = Build Array(w388, w388, w387, w387, w388) -> (w390:dbl[])
                              n303 = Build Array(w386, w385, w385, w386, w386) -> (w391:dbl[])
                              n304 = Bundle(w390, w391) -> (w389:cluster{dbl[], dbl[]})  [unwired: 1 in]
                            }
                          }
                        }
                        n305 = local write "轴承压装力位移曲线"(w376) -> ()
                      }
                      frame #1 {
                        n306 = Wait (ms)(milliseconds to wait=u32 200 ("等待时间（毫秒）")) -> ()  [unwired: 1 out]
                      }
                      frame #2 {
                        n307 = local read "判定框参数"() -> (w405:string[][])
                        n308 = Index Array(array=w405, index (row) #1=4 ("索引 (行)"), index (row) #2=5 ("索引 (行)"), index (row) #3=6 ("索引 (行)"), index (row) #4=7 ("索引 (行)")) -> (element #1=w413:string[], element #2=w412:string[], element #3=w411:string[], element #4=w410:string[])  [unwired: 4 in]
                        n309 = local read "轴承压装力位移曲线"() -> (w414:cluster{dbl[], dbl[]}[])
                        n310 = Index Array(array=w413, index=1 ("索引")) -> (element=w406:string)
                        n311 = Index Array(array=w412, index=1 ("索引")) -> (element=w407:string)
                        n312 = Index Array(array=w411, index=1 ("索引")) -> (element=w408:string)
                        n313 = Index Array(array=w410, index=1 ("索引")) -> (element=w409:string)
                        n314 = Fract/Exp String To Number(string=w406) -> (number=w404:dbl)  [unwired: 3 in, 1 out]
                        n315 = Fract/Exp String To Number(string=w407) -> (number=w403:dbl)  [unwired: 3 in, 1 out]
                        n316 = Fract/Exp String To Number(string=w408) -> (number=w402:dbl)  [unwired: 3 in, 1 out]
                        n317 = Fract/Exp String To Number(string=w409) -> (number=w401:dbl)  [unwired: 3 in, 1 out]
                        n318 = for {
                          tunnel: [w422] -> w415 mode=indexing
                          tunnel: w414 -> [w421] mode=indexing
                          tunnel: w404 -> [w419]
                          tunnel: w403 -> [w418]
                          tunnel: w402 -> [w417]
                          tunnel: w401 -> [w416]
                          i -> [w420]
                          n319 = case shown="1" w420 {
                            tunnel: [w423 w428] -> w422
                            tunnel: w421 -> [w423 _]
                            tunnel: w419 -> [_ w427]
                            tunnel: w418 -> [_ w426]
                            tunnel: w417 -> [_ w425]
                            tunnel: w416 -> [_ w424]
                            frame Default {
                            }
                            frame 1 {
                              n320 = Build Array(w427, w427, w426, w426, w427) -> (w429:dbl[])
                              n321 = Build Array(w425, w424, w424, w425, w425) -> (w430:dbl[])
                              n322 = Bundle(w429, w430) -> (w428:cluster{dbl[], dbl[]})  [unwired: 1 in]
                            }
                          }
                        }
                        n323 = local write "轴承压装力位移曲线"(w415) -> ()
                      }
                    }
                  }
                  frame 5 {
                    w432 = FALSE
                    w434 = u32 0
                    w435 = "" ("侧铆判定结果")
                    w433 = u16 0 ("备用_1")
                    w436 = nan ("侧铆最大压力(KN)")
                    n324 = shared-variable "我的电脑\\140轴承压装曲线.lvlib\\备用_1"(w433) -> ()  [unwired: 1 in, 1 out]
                    n325 = shared-variable "我的电脑\\140轴承压装曲线.lvlib\\备用_3"(w433) -> ()  [unwired: 1 in, 1 out]
                    n326 = shared-variable "我的电脑\\140轴承压装曲线.lvlib\\备用_4"(w433) -> ()  [unwired: 1 in, 1 out]
                    n327 = shared-variable "我的电脑\\140轴承压装曲线.lvlib\\备用_5"(w433) -> ()  [unwired: 1 in, 1 out]
                    n328 = shared-variable "我的电脑\\140轴承压装曲线.lvlib\\备用_6"(w433) -> ()  [unwired: 1 in, 1 out]
                    n329 = shared-variable "我的电脑\\140轴承压装曲线.lvlib\\备用_7"(w433) -> ()  [unwired: 1 in, 1 out]
                    n330 = local write "侧铆最大压力(KN)"(w436) -> ()
                    n331 = local write "端铆最大压力0°(KN)"(w436) -> ()
                    n332 = local write "端铆最大压力45°(KN)"(w436) -> ()
                    n333 = local write "侧铆判定结果"(w435) -> ()
                    n334 = local write "端铆判定结果0°"(w435) -> ()
                    n335 = local write "端铆判定结果45°"(w435) -> ()
                    n336 = local write "轴承压装判定结果"(bool[][] [] ("轴承压装判定结果")) -> ()
                    n337 = property on="侧铆最大压力(KN)" class="DigNum (严格)"("NumText.TextColor"=w434) -> ()  [unwired: 2 in, 2 out]
                    n338 = property on="端铆最大压力45°(KN)" class="DigNum (严格)"("NumText.TextColor"=w434) -> ()  [unwired: 2 in, 2 out]
                    n339 = property on="端铆最大压力0°(KN)" class="DigNum (严格)"("NumText.TextColor"=w434) -> ()  [unwired: 2 in, 2 out]
                    n340 = local write "不合格指示灯"(w432) -> ()
                    n341 = local write "合格指示灯"(w432) -> ()
                  }
                  frame 10 {
                    n342 = stacked-sequence {
                      frame #0 {
                        n343 = shared-variable "我的电脑\\140轴承压装曲线.lvlib\\压力传感器值"() -> (w448:sgl[])  [unwired: 1 in, 1 out]
                        n344 = local read "侧铆最大压力上限"() -> (w440:dbl)
                        n345 = local read "侧铆最大压力下限"() -> (w439:dbl)
                        n346 = Index Array(array=w448, index=0 ("索引")) -> (element=w437:sgl)
                        n347 = Greater?(x=w440, y=w437) -> (0:w446:bool)
                        n348 = Greater?(x=w437, y=w439) -> (0:w445:bool)
                        n349 = In Range and Coerce(upper limit=w440, x=w437, lower limit=w439) -> (In Range?=w438:bool)  [unwired: 1 out]
                        n350 = local write "侧铆最大压力(KN)"(w437) -> ()
                        n351 = And(x=w446, y=w445) -> (x .and. y?=w443:bool)
                        n352 = case shown="真" w438 {
                          frame False {
                            w449 = u32 16711680
                            n353 = property on="侧铆最大压力(KN)" class="DigNum (严格)"("NumText.TextColor"=w449) -> ()  [unwired: 2 in, 2 out]
                            n354 = property on="侧铆判定结果" class="Str"("Text.TextColor"=w449) -> ()  [unwired: 2 in, 2 out]
                            n355 = local write "侧铆判定结果"("NG" ("侧铆判定结果")) -> ()
                          }
                          frame True {
                            w452 = u32 46120
                            n356 = property on="侧铆最大压力(KN)" class="DigNum (严格)"("NumText.TextColor"=w452) -> ()  [unwired: 2 in, 2 out]
                            n357 = property on="侧铆判定结果" class="Str"("Text.TextColor"=w452) -> ()  [unwired: 2 in, 2 out]
                            n358 = local write "侧铆判定结果"("OK" ("侧铆判定结果")) -> ()
                          }
                        }
                        n359 = Not(x=w443) -> (.not. x?=w442:bool)
                        n360 = Build Array(w443, w442) -> (w444:bool[])
                        n361 = Boolean Array To Number(Boolean array=w444) -> (number=w441:u32)
                        n362 = shared-variable "我的电脑\\140轴承压装曲线.lvlib\\备用_4"(w441) -> ()  [unwired: 1 in, 1 out]
                      }
                      frame #1 {
                        n363 = Wait (ms)(milliseconds to wait=u32 800 ("等待时间（毫秒）")) -> ()  [unwired: 1 out]
                      }
                      frame #2 {
                        n364 = shared-variable "我的电脑\\140轴承压装曲线.lvlib\\备用_7"() -> (w454:u16)  [unwired: 1 in, 1 out]
                        n365 = case shown="0, 默认" w454 {
                          frame 0, Default {
                          }
                          frame 1 {
                            n366 = local write "合格指示灯"(TRUE ("合格指示灯")) -> ()
                            n367 = local write "不合格指示灯"(FALSE ("不合格指示灯")) -> ()
                          }
                          frame 2 {
                            n368 = local write "合格指示灯"(FALSE ("合格指示灯")) -> ()
                            n369 = local write "不合格指示灯"(TRUE ("不合格指示灯")) -> ()
                          }
                        }
                      }
                      frame #3 {
                        n370 = shared-variable "我的电脑\\140轴承压装曲线.lvlib\\备用_1"(100) -> ()  [unwired: 1 in, 1 out]
                      }
                    }
                  }
                  frame 20 {
                    n371 = stacked-sequence {
                      frame #0 {
                        n372 = shared-variable "我的电脑\\140轴承压装曲线.lvlib\\压力传感器值"() -> (w471:sgl[])  [unwired: 1 in, 1 out]
                        n373 = local read "端铆最大压力0°下限"() -> (w462:dbl)
                        n374 = local read "端铆最大压力0°上限"() -> (w463:dbl)
                        n375 = Index Array(array=w471, index=1 ("索引")) -> (element=w460:sgl)
                        n376 = local write "端铆最大压力0°(KN)"(w460) -> ()
                        n377 = Greater?(x=w463, y=w460) -> (0:w469:bool)
                        n378 = Greater?(x=w460, y=w462) -> (0:w468:bool)
                        n379 = In Range and Coerce(upper limit=w463, x=w460, lower limit=w462) -> (In Range?=w461:bool)  [unwired: 1 out]
                        n380 = And(x=w469, y=w468) -> (x .and. y?=w466:bool)
                        n381 = case shown="真" w461 {
                          frame False {
                            w472 = u32 16711680
                            n382 = property on="端铆判定结果0°" class="Str"("Text.TextColor"=w472) -> ()  [unwired: 2 in, 2 out]
                            n383 = property on="端铆最大压力0°(KN)" class="DigNum (严格)"("NumText.TextColor"=w472) -> ()  [unwired: 2 in, 2 out]
                            n384 = local write "端铆判定结果0°"("NG" ("侧铆判定结果")) -> ()
                          }
                          frame True {
                            w474 = u32 46120
                            n385 = property on="端铆判定结果0°" class="Str"("Text.TextColor"=w474) -> ()  [unwired: 2 in, 2 out]
                            n386 = property on="端铆最大压力0°(KN)" class="DigNum (严格)"("NumText.TextColor"=w474) -> ()  [unwired: 2 in, 2 out]
                            n387 = local write "端铆判定结果0°"("OK" ("侧铆判定结果")) -> ()
                          }
                        }
                        n388 = Not(x=w466) -> (.not. x?=w465:bool)
                        n389 = Build Array(w466, w465) -> (w467:bool[])
                        n390 = Boolean Array To Number(Boolean array=w467) -> (number=w464:u32)
                        n391 = shared-variable "我的电脑\\140轴承压装曲线.lvlib\\备用_5"(w464) -> ()  [unwired: 1 in, 1 out]
                      }
                      frame #1 {
                        n392 = Wait (ms)(milliseconds to wait=u32 800 ("等待时间（毫秒）")) -> ()  [unwired: 1 out]
                      }
                      frame #2 {
                        n393 = shared-variable "我的电脑\\140轴承压装曲线.lvlib\\备用_7"() -> (w477:u16)  [unwired: 1 in, 1 out]
                        n394 = case shown="2" w477 {
                          frame 0, Default {
                          }
                          frame 1 {
                            n395 = local write "合格指示灯"(TRUE ("合格指示灯")) -> ()
                            n396 = local write "不合格指示灯"(FALSE ("不合格指示灯")) -> ()
                          }
                          frame 2 {
                            n397 = local write "合格指示灯"(FALSE ("合格指示灯")) -> ()
                            n398 = local write "不合格指示灯"(TRUE ("不合格指示灯")) -> ()
                          }
                        }
                      }
                      frame #3 {
                        n399 = shared-variable "我的电脑\\140轴承压装曲线.lvlib\\备用_1"(100) -> ()  [unwired: 1 in, 1 out]
                      }
                    }
                    n400 = stacked-sequence {
                      frame #0 {
                        n401 = shared-variable "我的电脑\\140轴承压装曲线.lvlib\\压力传感器值"() -> (w494:sgl[])  [unwired: 1 in, 1 out]
                        n402 = local read "端铆最大压力0°下限"() -> (w484:dbl)
                        n403 = local read "端铆最大压力0°上限"() -> (w486:dbl)
                        n404 = Index Array(array=w494, index=1 ("索引")) -> (element=w485:sgl)
                        n405 = Greater?(x=w486, y=w485) -> (0:w492:bool)
                        n406 = Greater?(x=w485, y=w484) -> (0:w491:bool)
                        n407 = In Range and Coerce(upper limit=w486, x=w485, lower limit=w484) -> (In Range?=w483:bool)  [unwired: 1 out]
                        n408 = And(x=w492, y=w491) -> (x .and. y?=w489:bool)
                        n409 = case shown="假" w483 {
                          frame False {
                            w495 = u32 16711680
                            n410 = property on="端铆判定结果0°" class="Str"("Text.TextColor"=w495) -> ()  [unwired: 2 in, 2 out]
                            n411 = property on="端铆最大压力0°(KN)" class="DigNum (严格)"("NumText.TextColor"=w495) -> ()  [unwired: 2 in, 2 out]
                            n412 = flat-sequence {
                              tunnel: "NG" ("侧铆判定结果") -> [w497]
                              frame #0 {
                                n413 = local write "端铆判定结果0°"(w497) -> ()
                              }
                            }
                          }
                          frame True {
                            w498 = u32 46120
                            n414 = property on="端铆判定结果0°" class="Str"("Text.TextColor"=w498) -> ()  [unwired: 2 in, 2 out]
                            n415 = property on="端铆最大压力0°(KN)" class="DigNum (严格)"("NumText.TextColor"=w498) -> ()  [unwired: 2 in, 2 out]
                            n416 = local write "端铆判定结果0°"("OK" ("侧铆判定结果")) -> ()
                          }
                        }
                        n417 = Not(x=w489) -> (.not. x?=w488:bool)
                        n418 = Build Array(w489, w488) -> (w490:bool[])
                        n419 = Boolean Array To Number(Boolean array=w490) -> (number=w487:u32)
                        n420 = shared-variable "我的电脑\\140轴承压装曲线.lvlib\\备用_5"(w487) -> ()  [unwired: 1 in, 1 out]
                      }
                      frame #1 {
                        n421 = Wait (ms)(milliseconds to wait=u32 200 ("等待时间（毫秒）")) -> ()  [unwired: 1 out]
                      }
                      frame #2 {
                        n422 = shared-variable "我的电脑\\140轴承压装曲线.lvlib\\备用_2"() -> (w501:u16)  [unwired: 1 in, 1 out]
                        n423 = case shown="1" w501 {
                          frame 0, Default {
                          }
                          frame 1 {
                            n424 = shared-variable "我的电脑\\140轴承压装曲线.lvlib\\备用_5"() -> (w502:u16)  [unwired: 1 in, 1 out]
                            n425 = case shown="2" w502 {
                              frame 0, Default {
                              }
                              frame 1 {
                                n426 = local write "合格指示灯"(TRUE ("合格指示灯")) -> ()
                                n427 = local write "不合格指示灯"(FALSE ("不合格指示灯")) -> ()
                                n428 = shared-variable "我的电脑\\140轴承压装曲线.lvlib\\备用_7"(u16 1 ("备用_5")) -> ()  [unwired: 1 in, 1 out]
                              }
                              frame 2 {
                                n429 = local write "合格指示灯"(FALSE ("合格指示灯")) -> ()
                                n430 = local write "不合格指示灯"(TRUE ("不合格指示灯")) -> ()
                                n431 = shared-variable "我的电脑\\140轴承压装曲线.lvlib\\备用_7"(u16 2 ("备用_5")) -> ()  [unwired: 1 in, 1 out]
                              }
                            }
                          }
                          frame 2 {
                            n432 = shared-variable "我的电脑\\140轴承压装曲线.lvlib\\备用_4"() -> (w509:u16)  [unwired: 1 in, 1 out]
                            n433 = case shown="1" w509 {
                              frame 0, Default {
                              }
                              frame 1 {
                                n434 = shared-variable "我的电脑\\140轴承压装曲线.lvlib\\备用_7"(u16 2 ("备用_5")) -> ()  [unwired: 1 in, 1 out]
                                n435 = local write "合格指示灯"(FALSE ("合格指示灯")) -> ()
                                n436 = local write "不合格指示灯"(TRUE ("不合格指示灯")) -> ()
                              }
                              frame 2 {
                                n437 = shared-variable "我的电脑\\140轴承压装曲线.lvlib\\备用_7"(u16 2 ("备用_5")) -> ()  [unwired: 1 in, 1 out]
                                n438 = local write "合格指示灯"(FALSE ("合格指示灯")) -> ()
                                n439 = local write "不合格指示灯"(TRUE ("不合格指示灯")) -> ()
                              }
                            }
                          }
                        }
                      }
                    }
                  }
                  frame 30 {
                    n440 = stacked-sequence {
                      frame #0 {
                        n441 = shared-variable "我的电脑\\140轴承压装曲线.lvlib\\压力传感器值"() -> (w537:sgl[])  [unwired: 1 in, 1 out]
                        n442 = shared-variable "我的电脑\\140轴承压装曲线.lvlib\\压力传感器值"() -> (w529:sgl[])  [unwired: 1 in, 1 out]
                        n443 = local read "端铆最大压力45°上限"() -> (w520:dbl)
                        n444 = local read "端铆最大压力45°下限"() -> (w519:dbl)
                        n445 = local read "端铆最大压力0°下限"() -> (w521:dbl)
                        n446 = local read "端铆最大压力0°上限"() -> (w522:dbl)
                        n447 = Index Array(array=w537, index=1 ("索引")) -> (element=w517:sgl)
                        n448 = Index Array(array=w529, index=2 ("索引")) -> (element=w516:sgl)
                        n449 = local write "端铆最大压力0°(KN)"(w517) -> ()
                        n450 = local write "端铆最大压力45°(KN)"(w516) -> ()
                        n451 = Greater?(x=w520, y=w516) -> (0:w527:bool)
                        n452 = Greater?(x=w516, y=w519) -> (0:w526:bool)
                        n453 = Greater?(x=w522, y=w517) -> (0:w535:bool)
                        n454 = Greater?(x=w517, y=w521) -> (0:w534:bool)
                        n455 = And(x=w527, y=w526) -> (x .and. y?=w524:bool)
                        n456 = And(x=w535, y=w534) -> (x .and. y?=w525:bool)
                        n457 = In Range and Coerce(upper limit=w522, x=w517, lower limit=w521) -> (In Range?=w530:bool)  [unwired: 1 out]
                        n458 = In Range and Coerce(upper limit=w520, x=w516, lower limit=w519) -> (In Range?=w518:bool)  [unwired: 1 out]
                        n459 = And(x=w525, y=w524) -> (x .and. y?=w523:bool)
                        n460 = case shown="假" w518 {
                          frame False {
                            w538 = u32 16711680
                            n461 = property on="端铆最大压力45°(KN)" class="DigNum (严格)"("NumText.TextColor"=w538) -> ()  [unwired: 2 in, 2 out]
                            n462 = property on="端铆判定结果45°" class="Str"("Text.TextColor"=w538) -> ()  [unwired: 2 in, 2 out]
                            n463 = local write "端铆判定结果45°"("NG" ("端铆判定结果45°")) -> ()
                          }
                          frame True {
                            w540 = u32 46120
                            n464 = property on="端铆最大压力45°(KN)" class="DigNum (严格)"("NumText.TextColor"=w540) -> ()  [unwired: 2 in, 2 out]
                            n465 = property on="端铆判定结果45°" class="Str"("Text.TextColor"=w540) -> ()  [unwired: 2 in, 2 out]
                            n466 = local write "端铆判定结果45°"("OK" ("端铆判定结果45°")) -> ()
                          }
                        }
                        n467 = case shown="假" w530 {
                          frame False {
                            w542 = u32 16711680
                            n468 = property on="端铆判定结果0°" class="Str"("Text.TextColor"=w542) -> ()  [unwired: 2 in, 2 out]
                            n469 = property on="端铆最大压力0°(KN)" class="DigNum (严格)"("NumText.TextColor"=w542) -> ()  [unwired: 2 in, 2 out]
                            n470 = local write "端铆判定结果0°"("NG" ("侧铆判定结果")) -> ()
                          }
                          frame True {
                            w544 = u32 46120
                            n471 = property on="端铆判定结果0°" class="Str"("Text.TextColor"=w544) -> ()  [unwired: 2 in, 2 out]
                            n472 = property on="端铆最大压力0°(KN)" class="DigNum (严格)"("NumText.TextColor"=w544) -> ()  [unwired: 2 in, 2 out]
                            n473 = local write "端铆判定结果0°"("OK" ("侧铆判定结果")) -> ()
                          }
                        }
                        n474 = Not(x=w523) -> (.not. x?=w532:bool)
                        n475 = Build Array(w523, w532) -> (w533:bool[])
                        n476 = Boolean Array To Number(Boolean array=w533) -> (number=w531:u32)
                        n477 = shared-variable "我的电脑\\140轴承压装曲线.lvlib\\备用_6"(w531) -> ()  [unwired: 1 in, 1 out]
                      }
                      frame #1 {
                        n478 = Wait (ms)(milliseconds to wait=u32 800 ("等待时间（毫秒）")) -> ()  [unwired: 1 out]
                      }
                      frame #2 {
                        n479 = shared-variable "我的电脑\\140轴承压装曲线.lvlib\\备用_7"() -> (w547:u16)  [unwired: 1 in, 1 out]
                        n480 = case shown="2" w547 {
                          frame 0, Default {
                          }
                          frame 1 {
                            n481 = local write "合格指示灯"(TRUE ("合格指示灯")) -> ()
                            n482 = local write "不合格指示灯"(FALSE ("不合格指示灯")) -> ()
                          }
                          frame 2 {
                            n483 = local write "合格指示灯"(FALSE ("合格指示灯")) -> ()
                            n484 = local write "不合格指示灯"(TRUE ("不合格指示灯")) -> ()
                          }
                        }
                      }
                      frame #3 {
                        n485 = shared-variable "我的电脑\\140轴承压装曲线.lvlib\\备用_1"(100) -> ()  [unwired: 1 in, 1 out]
                      }
                    }
                  }
                  frame 100 {
                    n486 = stacked-sequence {
                      frame #0 {
                        w554 = "KN" ("元素")
                        w561 = "KN" ("元素")
                        n487 = local read "位移区间1内最大压力(KN)"() -> (w601:dbl)
                        n488 = local read "位移区间2内最小压力(KN)"() -> (w571:dbl)
                        n489 = local read "最大压力上限"() -> (w603:dbl)
                        n490 = local read "最大压力下限"() -> (w602:dbl)
                        n491 = local read "位移区间2内最大压力(KN)"() -> (w577:dbl)
                        n492 = local read "最小压力下限 2"() -> (w570:dbl)
                        n493 = local read "最小压力上限 2"() -> (w569:dbl)
                        n494 = local read "判定结果2 2"() -> (w559:string)
                        n495 = local read "判定结果1"() -> (w563:string)
                        n496 = local read "最大压力上限 2"() -> (w575:dbl)
                        n497 = local read "最大压力下限 2"() -> (w576:dbl)
                        n498 = Number To Fractional String(number=w601) -> (F-format string=w610:string)  [unwired: 3 in]
                        n499 = Number To Fractional String(number=w602) -> (F-format string=w611:string)  [unwired: 3 in]
                        n500 = Number To Fractional String(number=w603) -> (F-format string=w612:string)  [unwired: 3 in]
                        n501 = Number To Fractional String(number=w571) -> (F-format string=w568:string)  [unwired: 3 in]
                        n502 = Number To Fractional String(number=w570) -> (F-format string=w567:string)  [unwired: 3 in]
                        n503 = Number To Fractional String(number=w569) -> (F-format string=w566:string)  [unwired: 3 in]
                        n504 = local read "端铆判定结果45°"() -> (w553:string)
                        n505 = Number To Fractional String(number=w577) -> (F-format string=w574:string)  [unwired: 3 in]
                        n506 = Number To Fractional String(number=w576) -> (F-format string=w573:string)  [unwired: 3 in]
                        n507 = Number To Fractional String(number=w575) -> (F-format string=w572:string)  [unwired: 3 in]
                        n508 = shared-variable "我的电脑\\140轴承压装曲线.lvlib\\压力传感器值"() -> (w622:sgl[])  [unwired: 1 in, 1 out]
                        n509 = local read "端铆判定结果0°"() -> (w555:string)
                        n510 = local read "侧铆判定结果"() -> (w556:string)
                        n511 = Build Array(w610, w611, w612, w561, w563) -> (w620:string[])
                        n512 = local read "判定结果1 2"() -> (w560:string)
                        n513 = Build Array(w568, w567, w566, w561, w559) -> (w564:string[])
                        n514 = local read "判定结果3"() -> (w557:string)
                        n515 = local read "位移区间1内最小压力(KN)"() -> (w604:dbl)
                        n516 = local read "压装最终位移(mm)"() -> (w609:dbl)
                        n517 = local read "压装最终位移上限"() -> (w607:dbl)
                        n518 = local read "压装最终位移下限"() -> (w608:dbl)
                        n519 = local read "端铆最大压力45°下限"() -> (w586:dbl)
                        n520 = local read "端铆最大压力45°上限"() -> (w585:dbl)
                        n521 = local read "最小压力下限"() -> (w605:dbl)
                        n522 = local read "最小压力上限"() -> (w606:dbl)
                        n523 = local read "端铆最大压力0°下限"() -> (w591:dbl)
                        n524 = local read "端铆最大压力0°上限"() -> (w590:dbl)
                        n525 = Build Array(w574, w573, w572, w561, w560) -> (w565:string[])
                        n526 = local read "侧铆最大压力下限"() -> (w595:dbl)
                        n527 = local read "侧铆最大压力上限"() -> (w594:dbl)
                        n528 = Index Array(array=w622, index=2 ("索引")) -> (element=w587:sgl)
                        n529 = Index Array(array=w622, index=0 ("索引")) -> (element=w588:sgl)
                        n530 = Index Array(array=w622, index=1 ("索引")) -> (element=w589:sgl)
                        n531 = local read "判定结果2"() -> (w562:string)
                        n532 = Number To Fractional String(number=w604) -> (F-format string=w613:string)  [unwired: 3 in]
                        n533 = Number To Fractional String(number=w605) -> (F-format string=w614:string)  [unwired: 3 in]
                        n534 = Number To Fractional String(number=w606) -> (F-format string=w615:string)  [unwired: 3 in]
                        n535 = Number To Fractional String(number=w588) -> (F-format string=w623:string)  [unwired: 3 in]
                        n536 = Number To Fractional String(number=w595) -> (F-format string=w597:string)  [unwired: 3 in]
                        n537 = Number To Fractional String(number=w590) -> (F-format string=w592:string)  [unwired: 3 in]
                        n538 = Number To Fractional String(number=w587) -> (F-format string=w625:string)  [unwired: 3 in]
                        n539 = Number To Fractional String(number=w609) -> (F-format string=w616:string)  [unwired: 3 in]
                        n540 = Number To Fractional String(number=w608) -> (F-format string=w617:string)  [unwired: 3 in]
                        n541 = Number To Fractional String(number=w607) -> (F-format string=w618:string)  [unwired: 3 in]
                        n542 = Number To Fractional String(number=w594) -> (F-format string=w596:string)  [unwired: 3 in]
                        n543 = Number To Fractional String(number=w589) -> (F-format string=w624:string)  [unwired: 3 in]
                        n544 = Number To Fractional String(number=w591) -> (F-format string=w593:string)  [unwired: 3 in]
                        n545 = Number To Fractional String(number=w586) -> (F-format string=w584:string)  [unwired: 3 in]
                        n546 = Number To Fractional String(number=w585) -> (F-format string=w583:string)  [unwired: 3 in]
                        n547 = Build Array(w616, w617, w618, "mm" ("元素"), w557) -> (w581:string[])
                        n548 = Build Array(w623, w597, w596, w554, w556) -> (w580:string[])
                        n549 = Build Array(w613, w614, w615, w561, w562) -> (w619:string[])
                        n550 = Build Array(w624, w593, w592, w554, w555) -> (w579:string[])
                        n551 = Build Array(w625, w584, w583, w554, w553) -> (w578:string[])
                        n552 = Build Array(w620, w619, w565, w564, w581, w580, w579, w578) -> (w621:string[][])
                        n553 = shared-variable "我的电脑\\140轴承压装曲线.lvlib\\备用_3"(u16 1 ("备用1")) -> ()  [unwired: 1 in, 1 out]
                        n554 = local write "轴承压装报表"(w621) -> ()
                      }
                      frame #1 {
                        n555 = global read "Global1.vi" "联机模式"() -> (w626:enum16{"单机", "追溯"})
                        n556 = case shown="\"追溯\"" w626 {
                          frame "单机", Default {
                          }
                          frame "追溯" {
                            n557 = control-ref of="轴承压装报表"() -> (w635:refnum<vi>)
                            n558 = property class="Tbl (严格)"(reference=w635) -> (reference out=w634:refnum<vi>, "Row Headers[]"=w632:string[])  [unwired: 1 in, 1 out]
                            n559 = property class="Tbl (严格)"(reference=w634) -> ("Value"=w633:string[][])  [unwired: 1 in, 2 out]
                            n560 = for {
                              tunnel: w633 -> [w638] mode=indexing
                              tunnel: w632 -> [w639] mode=indexing
                              tunnel: [w637] -> w631 mode=indexing if=w636
                              n561 = Index Array(array=w638) -> (element=w640:string)  [unwired: 1 in]
                              n562 = Build Array (concatenate)(w639, w638) -> (w637:string[])
                              n563 = case shown="默认" w640 {
                                tunnel: [TRUE FALSE] -> w636
                                frame Default {
                                }
                                frame "" {
                                }
                              }
                            }
                            n564 = local read "deviceid"() -> (w630:string)
                            n565 = local read "codeid"() -> (w628:string)
                            n566 = global read "追溯全部变量.vi" "工件状态"() -> (w627:string)
                            n567 = local read "USER_ID"() -> (w629:string)
                            n568 = call "UPTEST.vi"("Result"=w631, "CODE_ID"=w628, "DEVICE_ID"=w630) -> ()  [unwired: 6 in, 1 out]
                            n569 = call "UPRESULT.vi"("DEVICE_ID"=w630, "USER_ID"=w629, "CODE_ID"=w628, "RESULT_VALUE"=w627) -> ()  [unwired: 11 in, 1 out]
                          }
                        }
                      }
                      frame #2 {
                        n570 = Wait (ms)(milliseconds to wait=u32 50 ("等待时间（毫秒）")) -> ()  [unwired: 1 out]
                        n571 = call "浮动通知.vi"("通知内容"="报表生成中" ("Status")) -> ()  [unwired: 11 in]
                        n572 = control-ref of="轴承压装报表"() -> (w644:refnum<vi>)
                        n573 = control-ref of="轴承压装力位移曲线"() -> (w645:refnum<vi>)
                        n574 = global write "A131258.vi" "轴承压装力位移曲线"(w645) -> ()
                        n575 = global write "Global.vi" "轴承压装报表"(w644) -> ()
                        n576 = shared-variable "我的电脑\\140轴承压装曲线.lvlib\\备用_7"() -> (w643:u16)  [unwired: 1 in, 1 out]
                        n577 = case shown="1" w643 {
                          frame 0, Default {
                          }
                          frame 1 {
                            n578 = local write "不合格指示灯"(FALSE ("不合格指示灯")) -> ()
                            n579 = local write "合格指示灯"(TRUE ("合格指示灯")) -> ()
                            n580 = local write "轴承压装判定结果"(bool[][] [[TRUE, TRUE]] ("判定结果")) -> ()
                          }
                          frame 2 {
                            n581 = local write "不合格指示灯"(TRUE ("不合格指示灯")) -> ()
                            n582 = local write "合格指示灯"(FALSE ("合格指示灯")) -> ()
                            n583 = local write "轴承压装判定结果"(bool[][] [[TRUE, FALSE]] ("判定结果")) -> ()
                          }
                        }
                        n584 = shared-variable "我的电脑\\140轴承压装曲线.lvlib\\备用_1"(u16 101 ("备用1")) -> ()  [unwired: 1 in, 1 out]
                      }
                    }
                  }
                  frame 101 {
                    n585 = stacked-sequence {
                      frame #0 {
                        n586 = global read "Global1.vi" "联机模式"() -> (w655:enum16{"单机", "追溯"})
                        n587 = case shown="\"追溯\"" w655 {
                          frame "单机", Default {
                            n588 = shared-variable "我的电脑\\140轴承压装曲线.lvlib\\备用_1"(u16 102 ("备用1")) -> ()  [unwired: 1 in, 1 out]
                          }
                          frame "追溯" {
                            n589 = disable-structure shown="禁用" {
                              frame Disabled {
                                n590 = local read "产品条码"() -> (w662:string)
                                n591 = global read "Global1.vi" "联机模式"() -> (w670:enum16{"单机", "追溯"})
                                n592 = local read "productid"() -> (w665:string)
                                n593 = call "GetSQLstring.vi"("联机模式"=w670) -> ("错误输出"=w672:errorcluster, "连接字符串"=w671:string)  [unwired: 9 in]
                                n594 = call-poly <vilib>:"DB Tools Open Connection.vi"("error in (no error)"=w672, "connection information"=w671) -> ("error out"=w678:errorcluster, "connection reference"=w677:T5)  [unwired: 6 in]
                                n595 = Concatenate Strings("SELECT CODE_ID FROM [Code]  WHERE CODE_MAIN ='" ("字符串"), w662, "'", " AND PRODUCT_ID='" ("字符串"), w665, "'" ("字符串")) -> (w673:string)
                                n596 = call-poly <vilib>:"DB Tools Execute Query.vi"("error in (no error)"=w678, "SQL query"=w673, "connection reference"=w677) -> ("error out"=w675:errorcluster, "recordset reference"=w674:T6)  [unwired: 5 in]
                                n597 = call-poly <vilib>:"DB Tools Fetch Recordset Data.vi"("error in (no error)"=w675, "recordset reference"=w674) -> ("error out"=w679:errorcluster, "recordset data"=w676:variant[][])  [unwired: 3 in, 1 out]
                                n598 = Variant To Data(error in=w679, type=string[][] [], Variant=w676) -> (data=w680:string[][], error out=w660:errorcluster)
                                n599 = Index Array(array=w680, index (row)=0 ("索引 (行)")) -> (element=w681:string[])  [unwired: 1 in]
                                n600 = call <vilib>:"Simple Error Handler.vi"("error in (no error)"=w660) -> ()  [unwired: 4 in, 5 out]
                                n601 = Index Array(array=w681, index=0 ("索引 (行)")) -> ()  [unwired: 1 out]
                              }
                              frame Enabled {
                              }
                            }
                            n602 = local read "产品条码"() -> (w659:string)
                            n603 = local read "productid"() -> (w657:string)
                            n604 = call "Get_CODE_ID.vi"("PRODUCT_ID"=w657, "CODE_MAIN"=w659) -> ("CODE_ID"=→"codeid":string)  [unwired: 9 in]
                          }
                        }
                      }
                      frame #1 {
                        n605 = local read "合格指示灯"() -> (w683:bool)
                        n606 = local read "产品条码"() -> (w682:string)
                        n607 = call "Report_A131258.vi"("文件重命名"=TRUE, "文件名称"=w682, "合格状态"=w683, "布尔数组"="轴承压装判定结果") -> ()  [unwired: 7 in, 1 out]
                      }
                      frame #2 {
                        n608 = shared-variable "我的电脑\\140轴承压装曲线.lvlib\\备用_1"(u16 102 ("备用1")) -> ()  [unwired: 1 in, 1 out]
                      }
                    }
                  }
                  frame 102 {
                    n609 = shared-variable "我的电脑\\140轴承压装曲线.lvlib\\备用_1"(u16 103 ("备用1")) -> ()  [unwired: 1 in, 1 out]
                  }
                  frame 103 {
                    n610 = global read "Global1.vi" "联机模式"() -> (w688:enum16{"单机", "追溯"})
                    n611 = case shown="\"追溯\"" w688 {
                      tunnel: w688 -> [_ w691]
                      frame "单机", Default {
                        n612 = shared-variable "我的电脑\\140轴承压装曲线.lvlib\\备用_3"(u16 0 ("备用1")) -> ()  [unwired: 1 in, 1 out]
                        n613 = shared-variable "我的电脑\\140轴承压装曲线.lvlib\\备用_1"(u16 0 ("备用1")) -> ()  [unwired: 1 in, 1 out]
                      }
                      frame "追溯" {
                        n614 = stacked-sequence {
                          tunnel: w691 -> [w692 _]
                          frame #0 {
                            n615 = disable-structure shown="禁用" {
                              disable-tunnel: w692 -> [w693 _]
                              frame Disabled {
                                n616 = shared-variable "我的电脑\\140轴承压装曲线.lvlib\\备用_7"() -> (w694:u16)  [unwired: 1 in, 1 out]
                                n617 = case shown="2" w694 {
                                tunnel: ["" "OK" "NG"] -> w695
                                frame 0, Default {
                                }
                                frame 1 {
                                }
                                frame 2 {
                                }
                                }
                                n618 = Get Date/Time String(date format (0)=enum16{"short", "long", "abbreviated"}."short" ("日期格式(0)"), want seconds? (F)=FALSE ("需要秒？(F)")) -> (date string=w706:string, time string=w705:string)  [unwired: 1 in]
                                n619 = local read "deviceid"() -> (w714:string)
                                n620 = local read "USER_ID"() -> (w697:string)
                                n621 = local read "codeid"() -> (w711:string)
                                n622 = Concatenate Strings(w706, " " ("字符串"), w705) -> (w702:string)
                                n623 = Decimal String To Number(string=w714, default (0L)=i64 0 ("默认(0 I32)")) -> (number=w712:i64)  [unwired: 1 in, 1 out]
                                n624 = Decimal String To Number(string=w697, default (0L)=i64 0 ("默认(0 I32)")) -> (number=w696:i64)  [unwired: 1 in, 1 out]
                                n625 = Decimal String To Number(string=w711, default (0L)=i64 0 ("默认(0 I32)")) -> (number=w709:i64)  [unwired: 1 in, 1 out]
                                n626 = Search and Replace String(replace all?=TRUE ("替换全部？(F)"), input string=w702, search string="/" ("替换字符串(\"\")"), replace string="-" ("替换字符串(\"\")")) -> (result string=w703:string)  [unwired: 4 in, 3 out]
                                n627 = Bundle(w712, w696, w709, w695, "result string"=w703) -> (w716:T7)  [unwired: 1 in]
                                n628 = call "GetSQLstring.vi"("联机模式"=w693) -> ("错误输出"=w719:errorcluster, "连接字符串"=w720:string)  [unwired: 9 in]
                                n629 = Build Array(w716) -> (w715:T8)
                                n630 = call-poly <vilib>:"DB Tools Open Connection.vi"("error in (no error)"=w719, "connection information"=w720) -> ("error out"=w721:errorcluster, "connection reference"=w718:T5)  [unwired: 6 in]
                                n631 = for {
                                tunnel: w715 -> [w729] mode=indexing
                                tunnel: w718 -> [w727]
                                shift-right: [w725] -> w717
                                shift-left: w721 -> [w732]
                                w728 = string[] ["DEVICE_ID", "USER_ID", "CODE_ID", "RESULT_VALUE", "RESULT_TIME"] ("columns")
                                w730 = "Result" ("table")
                                n632 = call <vilib>:"DB Tools Insert Data.vi"("data"=w729, "error in (no error)"=w732, "columns"=w728, "table"=w730, "connection reference"=w727) -> ("error out"=w731:errorcluster, "connection reference out"=w726:T5)  [unwired: 5 in]
                                n633 = case shown="错误" w731 {
                                selector: w731 -> [w733 w754]
                                tunnel: w728 -> [_ w751]
                                tunnel: w726 -> [w734 w741]
                                tunnel: w730 -> [_ w755]
                                tunnel: w729 -> [_ w745]
                                tunnel: [w734 w740] -> _
                                tunnel: [w733 w739] -> w725
                                frame No Error {
                                }
                                frame Error {
                                n634 = Array Subset(array=w751, index=3 ("长度"), length=2 ("索引")) -> (w752:string[])
                                n635 = Unbundle(w745) -> (w736:i64, w737:i64, w744:string, "result string"=w743:string)  [unwired: 1 out]
                                n636 = Bundle(w744, "result string"=w743) -> (w742:cluster{string, "result string":string})  [unwired: 1 in]
                                n637 = Number To Decimal String(number=w737) -> (decimal integer string=w738:string)  [unwired: 1 in]
                                n638 = call <vilib>:"Clear Errors.vi"("error in (no error)"=w754) -> ("error out"=w753:errorcluster)  [unwired: 5 in, 1 out]
                                n639 = Number To Decimal String(number=w736) -> (decimal integer string=w735:string)  [unwired: 1 in]
                                n640 = Concatenate Strings("WHERE CODE_ID =" ("condition"), w738, "AND DEVICE_ID =", w735) -> (w747:string)
                                n641 = call <vilib>:"DB Tools Update Data.vi"("condition"=w747, "data"=w742, "error in (no error)"=w753, "columns"=w752, "table"=w755, "connection reference"=w741) -> ("error out"=w739:errorcluster, "connection reference out"=w740:T5)  [unwired: 4 in]
                                }
                                }
                                }
                                n642 = call <vilib>:"Simple Error Handler.vi"("error in (no error)"=w717) -> ()  [unwired: 4 in, 5 out]
                              }
                              frame Enabled {
                              }
                            }
                          }
                          frame #1 {
                            n643 = shared-variable "我的电脑\\140轴承压装曲线.lvlib\\备用_3"(u16 0 ("备用1")) -> ()  [unwired: 1 in, 1 out]
                            n644 = shared-variable "我的电脑\\140轴承压装曲线.lvlib\\备用_1"(u16 0 ("备用1")) -> ()  [unwired: 1 in, 1 out]
                          }
                        }
                      }
                    }
                  }
                  frame 1000 {
                    n645 = stacked-sequence {
                      frame #0 {
                        n646 = Wait (ms)(milliseconds to wait=u32 300 ("等待时间（毫秒）")) -> ()  [unwired: 1 out]
                        n647 = shared-variable "我的电脑\\Global.lvlib\\工位追溯码"("" ("传感器码")) -> ()  [unwired: 1 in, 1 out]
                      }
                      frame #1 {
                        w761 = "请扫码！" ("通知内容")
                        n648 = call "浮动通知.vi"("通知内容"=w761) -> ()  [unwired: 11 in]
                        n649 = call "输入框.vi"("提示信息"=w761) -> ("条形码输出"=w762:string)
                        "产品条码" <- w762
                        n650 = shared-variable "我的电脑\\140轴承压装曲线.lvlib\\备用_1"(u16 1001 ("备用1")) -> ()  [unwired: 1 in, 1 out]
                        n651 = shared-variable "我的电脑\\Global.lvlib\\工位追溯码"(w762) -> ()  [unwired: 1 in, 1 out]
                      }
                    }
                  }
                  frame 1001 {
                    n652 = shared-variable "我的电脑\\Global.lvlib\\工位追溯码"() -> (w763:string)  [unwired: 1 in, 1 out]
                    n653 = String Length(string=w763) -> (length=w765:i32)
                    n654 = Greater?(x=w765, y=4) -> (0:w766:bool)
                    n655 = case shown="真" w766 {
                      frame False {
                      }
                      frame True {
                        n656 = shared-variable "我的电脑\\140轴承压装曲线.lvlib\\备用_1"(u16 1002 ("备用1")) -> ()  [unwired: 1 in, 1 out]
                      }
                    }
                  }
                }
              }
            }
          }
          event "删除": Value Change {
            n657 = event-data() -> ("NewVal"=w768:bool)  [unwired: 1 in, 5 out]
            n658 = case shown="真" w768 {
              tunnel: w769 -> [_ w771]
              frame False {
              }
              frame True {
                n659 = Concatenate Strings("确认删除“", "请选择要删除的产品", "”吗？") -> (w773:string)
                n660 = Two Button Dialog(message=w773) -> (T button?=w772:bool)  [unwired: 2 in]
                n661 = case shown="真" w772 {
                  tunnel: w771 -> [_ w777]
                  tunnel: "请选择要删除的产品" -> [_ w776]
                  frame False {
                  }
                  frame True {
                    n662 = call <vilib>:"Open Config Data.vi"("configuration file path"=w777) -> ("error out"=w779:errorcluster, "refnum"=w782:T4)  [unwired: 8 in, 1 out]
                    n663 = call <vilib>:"Remove Section.vi"("section"=w776, "error in (no error)"=w779, "refnum"=w782) -> ("error out"=w781:errorcluster, "section exists?"=w778:bool, "refnum out"=w780:T4)  [unwired: 6 in]
                    n664 = call <vilib>:"Close Config Data.vi"("error in (no error)"=w781, "refnum"=w780) -> ()  [unwired: 8 in, 2 out]
                    n665 = case shown="真" w778 {
                      frame False {
                        n666 = One Button Dialog(message="删除失败！\n请确认产品存在！" ("消息")) -> ()  [unwired: 1 in, 1 out]
                      }
                      frame True {
                        n667 = One Button Dialog(message="删除成功！" ("消息")) -> ()  [unwired: 1 in, 1 out]
                      }
                    }
                  }
                }
              }
            }
          }
          event "确定": Value Change {
            n668 = event-data() -> ("NewVal"=w785:bool)  [unwired: 1 in, 5 out]
            n669 = case shown="真" w785 {
              frame False {
              }
              frame True {
                n670 = stacked-sequence {
                  seq-local: [w789 _ _ _ _ _ _ _] -> [_ _ _ _ _ _ _ _]
                  frame #0 {
                    n671 = global read "Global1.vi" "联机模式"() -> (w786:enum16{"单机", "追溯"})
                    n672 = case shown="\"追溯\"" w786 {
                      frame "单机", Default {
                      }
                      frame "追溯" {
                        n673 = local read "产品型号"() -> (w792:string)
                        n674 = call "GET_PRODUCT_ID.vi"("PRODFUCT_NAME"=w792) -> ("PRODUCT_ID"=→"productid":string)  [unwired: 10 in]
                        n675 = call "Get_Device_ID.vi"() -> ("Device_ID"=→"deviceid":string)  [unwired: 10 in, 1 out]
                      }
                    }
                    n676 = property on="选项卡控件 2" class="TabCtl (严格)"("Value"=enum32{"轴承压装力位移曲线", "参数查看"}."轴承压装力位移曲线" ("选项卡控件 2")) -> ()  [unwired: 2 in, 2 out]
                    n677 = local read "产品型号"() -> (w788:string)
                    "产品型号" <- w788
                    n678 = shared-variable "我的电脑\\Global.lvlib\\产品型号"(w788) -> ()  [unwired: 1 in, 1 out]
                    n679 = String Subset(string=w788, offset (0)=u16 2 ("偏移量(0)"), length (rest)=u16 4 ("长度（剩余）")) -> (substring=w789:string)
                  }
                  frame #1 {
                    n680 = global read "Global1.vi" "联机模式"() -> (w795:enum16{"单机", "追溯"})
                    n681 = case shown="\"追溯\"" w795 {
                      frame "单机", Default {
                      }
                      frame "追溯" {
                        n682 = local read "用户名"() -> (w797:string)
                        n683 = global read "Global1.vi" "联机模式"() -> (w803:enum16{"单机", "追溯"})
                        n684 = call "GetSQLstring.vi"("联机模式"=w803) -> ("错误输出"=w805:errorcluster, "连接字符串"=w804:string)  [unwired: 9 in]
                        n685 = call-poly <vilib>:"DB Tools Open Connection.vi"("error in (no error)"=w805, "connection information"=w804) -> ("error out"=w811:errorcluster, "connection reference"=w810:T5)  [unwired: 6 in]
                        n686 = Concatenate Strings("SELECT USER_ID FROM [User]  WHERE USER_NAME ='" ("字符串"), w797, "'" ("字符串")) -> (w806:string)
                        n687 = call-poly <vilib>:"DB Tools Execute Query.vi"("error in (no error)"=w811, "SQL query"=w806, "connection reference"=w810) -> ("error out"=w808:errorcluster, "recordset reference"=w807:T6)  [unwired: 5 in]
                        n688 = call-poly <vilib>:"DB Tools Fetch Recordset Data.vi"("error in (no error)"=w808, "recordset reference"=w807) -> ("error out"=w812:errorcluster, "recordset data"=w809:variant[][])  [unwired: 3 in, 1 out]
                        n689 = Variant To Data(error in=w812, type=string[][] [], Variant=w809) -> (data=w813:string[][])  [unwired: 1 out]
                        n690 = Index Array(array=w813, index (row)=0 ("索引 (行)")) -> (element=w814:string[])  [unwired: 1 in]
                        n691 = Index Array(array=w814, index=0 ("索引 (行)")) -> (element=→"USER_ID":string)
                      }
                    }
                  }
                  frame #2 {
                    n692 = local read "坐标轴参数"() -> (w819:string[][])
                    n693 = Index Array(array=w819, index (row) #1=0 ("索引 (行)"), index (row) #2=1 ("索引 (行)"), index (row) #3=2 ("索引 (行)"), index (row) #4=3 ("索引 (行)")) -> (element #1=w831:string[], element #2=w826:string[], element #3=w825:string[], element #4=w824:string[])  [unwired: 4 in]
                    n694 = Index Array(array=w831, index=1 ("索引")) -> (element=w823:string)
                    n695 = Index Array(array=w826, index=1 ("索引")) -> (element=w822:string)
                    n696 = Index Array(array=w825, index=1 ("索引")) -> (element=w821:string)
                    n697 = Index Array(array=w824, index=1 ("索引")) -> (element=w820:string)
                    n698 = Fract/Exp String To Number(string=w823) -> (number=w818:dbl)  [unwired: 3 in, 1 out]
                    n699 = Fract/Exp String To Number(string=w822) -> (number=w817:dbl)  [unwired: 3 in, 1 out]
                    n700 = Fract/Exp String To Number(string=w821) -> (number=w816:dbl)  [unwired: 3 in, 1 out]
                    n701 = Fract/Exp String To Number(string=w820) -> (number=w815:dbl)  [unwired: 3 in, 1 out]
                    n702 = property on="轴承压装力位移曲线" class="XYGraph (严格)"("XScale.Minimum"=w818) -> ()  [unwired: 2 in, 2 out]
                    n703 = property on="轴承压装力位移曲线" class="XYGraph (严格)"("XScale.Maximum"=w817) -> ()  [unwired: 2 in, 2 out]
                    n704 = property on="轴承压装力位移曲线" class="XYGraph (严格)"("YScale.Minimum"=w816) -> ()  [unwired: 2 in, 2 out]
                    n705 = property on="轴承压装力位移曲线" class="XYGraph (严格)"("YScale.Maximum"=w815) -> ()  [unwired: 2 in, 2 out]
                  }
                  frame #3 {
                    n706 = local read "判定框参数"() -> (w845:string[][])
                    n707 = Index Array(array=w845, index (row) #1=0 ("索引 (行)"), index (row) #2=1 ("索引 (行)"), index (row) #3=2 ("索引 (行)"), index (row) #4=3 ("索引 (行)")) -> (element #1=w853:string[], element #2=w848:string[], element #3=w847:string[], element #4=w846:string[])  [unwired: 4 in]
                    n708 = local read "轴承压装力位移曲线"() -> (w858:cluster{dbl[], dbl[]}[])
                    n709 = Index Array(array=w853, index=1 ("索引")) -> (element=w840:string)
                    n710 = Index Array(array=w848, index=1 ("索引")) -> (element=w839:string)
                    n711 = Index Array(array=w847, index=1 ("索引")) -> (element=w838:string)
                    n712 = Index Array(array=w846, index=1 ("索引")) -> (element=w837:string)
                    n713 = Fract/Exp String To Number(string=w840) -> (number=w844:dbl)  [unwired: 3 in, 1 out]
                    n714 = Fract/Exp String To Number(string=w839) -> (number=w843:dbl)  [unwired: 3 in, 1 out]
                    n715 = Fract/Exp String To Number(string=w838) -> (number=w841:dbl)  [unwired: 3 in, 1 out]
                    n716 = Fract/Exp String To Number(string=w837) -> (number=w842:dbl)  [unwired: 3 in, 1 out]
                    n717 = for {
                      tunnel: [w865] -> w836 mode=indexing
                      tunnel: w858 -> [w864] mode=indexing
                      tunnel: w844 -> [w862]
                      tunnel: w843 -> [w861]
                      tunnel: w842 -> [w860]
                      tunnel: w841 -> [w859]
                      i -> [w863]
                      n718 = case shown="0" w863 {
                        tunnel: [w866 w871] -> w865
                        tunnel: w864 -> [w866 _]
                        tunnel: w862 -> [_ w870]
                        tunnel: w861 -> [_ w869]
                        tunnel: w860 -> [_ w868]
                        tunnel: w859 -> [_ w867]
                        frame Default {
                        }
                        frame 0 {
                          n719 = Build Array(w870, w870, w869, w869, w870) -> (w872:dbl[])
                          n720 = Build Array(w867, w868, w868, w867, w867) -> (w873:dbl[])
                          n721 = Bundle(w872, w873) -> (w871:cluster{dbl[], dbl[]})  [unwired: 1 in]
                        }
                      }
                    }
                    n722 = local write "轴承压装力位移曲线"(w836) -> ()
                  }
                  frame #4 {
                    n723 = Wait (ms)(milliseconds to wait=u32 200 ("等待时间（毫秒）")) -> ()  [unwired: 1 out]
                  }
                  frame #5 {
                    n724 = local read "判定框参数"() -> (w888:string[][])
                    n725 = Index Array(array=w888, index (row) #1=4 ("索引 (行)"), index (row) #2=5 ("索引 (行)"), index (row) #3=6 ("索引 (行)"), index (row) #4=7 ("索引 (行)")) -> (element #1=w884:string[], element #2=w885:string[], element #3=w886:string[], element #4=w887:string[])  [unwired: 4 in]
                    n726 = local read "轴承压装力位移曲线"() -> (w883:cluster{dbl[], dbl[]}[])
                    n727 = Index Array(array=w884, index=1 ("索引")) -> (element=w893:string)
                    n728 = Index Array(array=w885, index=1 ("索引")) -> (element=w894:string)
                    n729 = Index Array(array=w886, index=1 ("索引")) -> (element=w895:string)
                    n730 = Index Array(array=w887, index=1 ("索引")) -> (element=w896:string)
                    n731 = Fract/Exp String To Number(string=w893) -> (number=w889:dbl)  [unwired: 3 in, 1 out]
                    n732 = Fract/Exp String To Number(string=w894) -> (number=w890:dbl)  [unwired: 3 in, 1 out]
                    n733 = Fract/Exp String To Number(string=w895) -> (number=w892:dbl)  [unwired: 3 in, 1 out]
                    n734 = Fract/Exp String To Number(string=w896) -> (number=w891:dbl)  [unwired: 3 in, 1 out]
                    n735 = for {
                      tunnel: [w904] -> w897 mode=indexing
                      tunnel: w883 -> [w903] mode=indexing
                      tunnel: w889 -> [w901]
                      tunnel: w890 -> [w900]
                      tunnel: w891 -> [w899]
                      tunnel: w892 -> [w898]
                      i -> [w902]
                      n736 = case shown="1" w902 {
                        tunnel: [w905 w910] -> w904
                        tunnel: w903 -> [w905 _]
                        tunnel: w901 -> [_ w909]
                        tunnel: w900 -> [_ w908]
                        tunnel: w899 -> [_ w907]
                        tunnel: w898 -> [_ w906]
                        frame Default {
                        }
                        frame 1 {
                          n737 = Build Array(w909, w909, w908, w908, w909) -> (w911:dbl[])
                          n738 = Build Array(w906, w907, w907, w906, w906) -> (w912:dbl[])
                          n739 = Bundle(w911, w912) -> (w910:cluster{dbl[], dbl[]})  [unwired: 1 in]
                        }
                      }
                    }
                    n740 = local write "轴承压装力位移曲线"(w897) -> ()
                  }
                  frame #6 {
                    n741 = local read "判定框参数"() -> (w921:string[][])
                    n742 = local read "判定框参数"() -> (w956:string[][])
                    n743 = Index Array(array=w921, index (row) #1=6 ("索引 (行)"), index (row) #2=7 ("索引 (行)")) -> (element #1=w915:string[], element #2=w917:string[])  [unwired: 2 in]
                    n744 = Index Array(array=w956, index (row) #1=2 ("索引 (行)"), index (row) #2=3 ("索引 (行)")) -> (element #1=w973:string[], element #2=w971:string[])  [unwired: 2 in]
                    n745 = Index Array(array=w915, index=1 ("索引")) -> (element=w919:string)
                    n746 = Index Array(array=w917, index=1 ("索引")) -> (element=w920:string)
                    n747 = Index Array(array=w973, index=1 ("索引")) -> (element=w969:string)
                    n748 = Index Array(array=w971, index=1 ("索引")) -> (element=w968:string)
                    n749 = Fract/Exp String To Number(string=w919) -> (number=w923:dbl)  [unwired: 3 in, 1 out]
                    n750 = Fract/Exp String To Number(string=w920) -> (number=w922:dbl)  [unwired: 3 in, 1 out]
                    n751 = Fract/Exp String To Number(string=w969) -> (number=w954:dbl)  [unwired: 3 in, 1 out]
                    n752 = Fract/Exp String To Number(string=w968) -> (number=w955:dbl)  [unwired: 3 in, 1 out]
                    n753 = local write "最大压力下限"(w954) -> ()
                    n754 = local write "最小压力下限"(w954) -> ()
                    n755 = local write "最大压力上限"(w955) -> ()
                    n756 = local write "最小压力上限"(w955) -> ()
                    n757 = local write "最大压力下限 2"(w923) -> ()
                    n758 = local write "最小压力下限 2"(w923) -> ()
                    n759 = local write "最大压力上限 2"(w922) -> ()
                    n760 = local write "最小压力上限 2"(w922) -> ()
                    n761 = local read "结果判定参数"() -> (w959:string[][])
                    n762 = Index Array(array=w959, index (row) #1=0 ("索引 (行)"), index (row) #2=0 ("索引 (行)"), index (row) #3=1 ("索引 (行)"), index (row) #4=1 ("索引 (行)"), index (row) #5=2 ("索引 (行)"), index (row) #6=2 ("索引 (行)"), index (row) #7=3 ("索引 (行)"), index (row) #8=3 ("索引 (行)")) -> (element #1=w965:string[], element #2=w963:string[], element #3=w941:string[], element #4=w940:string[], element #5=w939:string[], element #6=w938:string[], element #7=w937:string[], element #8=w936:string[])  [unwired: 8 in]
                    n763 = Index Array(array=w965, index=1 ("索引")) -> (element=w961:string)
                    n764 = Index Array(array=w963, index=2 ("索引")) -> (element=w960:string)
                    n765 = Index Array(array=w941, index=1 ("索引")) -> (element=w935:string)
                    n766 = Index Array(array=w940, index=2 ("索引")) -> (element=w934:string)
                    n767 = Index Array(array=w939, index=1 ("索引")) -> (element=w933:string)
                    n768 = Index Array(array=w938, index=2 ("索引")) -> (element=w932:string)
                    n769 = Index Array(array=w937, index=1 ("索引")) -> (element=w931:string)
                    n770 = Index Array(array=w936, index=2 ("索引")) -> (element=w930:string)
                    n771 = Fract/Exp String To Number(string=w961) -> (number=w957:dbl)  [unwired: 3 in, 1 out]
                    n772 = Fract/Exp String To Number(string=w960) -> (number=w958:dbl)  [unwired: 3 in, 1 out]
                    n773 = Fract/Exp String To Number(string=w935) -> (number=w929:dbl)  [unwired: 3 in, 1 out]
                    n774 = Fract/Exp String To Number(string=w934) -> (number=w928:dbl)  [unwired: 3 in, 1 out]
                    n775 = Fract/Exp String To Number(string=w933) -> (number=w927:dbl)  [unwired: 3 in, 1 out]
                    n776 = Fract/Exp String To Number(string=w932) -> (number=w926:dbl)  [unwired: 3 in, 1 out]
                    n777 = Fract/Exp String To Number(string=w931) -> (number=w925:dbl)  [unwired: 3 in, 1 out]
                    n778 = Fract/Exp String To Number(string=w930) -> (number=w924:dbl)  [unwired: 3 in, 1 out]
                    n779 = local write "压装最终位移下限"(w957) -> ()
                    n780 = local write "压装最终位移上限"(w958) -> ()
                    n781 = local write "侧铆最大压力下限"(w929) -> ()
                    n782 = local write "侧铆最大压力上限"(w928) -> ()
                    n783 = local write "端铆最大压力0°下限"(w927) -> ()
                    n784 = local write "端铆最大压力0°上限"(w926) -> ()
                    n785 = local write "端铆最大压力45°下限"(w925) -> ()
                    n786 = local write "端铆最大压力45°上限"(w924) -> ()
                  }
                  frame #7 {
                    w976 = "参数装载成功！" ("消息")
                    n787 = One Button Dialog(message=w976) -> ()  [unwired: 1 in, 1 out]
                    n788 = call "浮动通知.vi"("通知内容"=w976) -> ()  [unwired: 11 in]
                  }
                }
              }
            }
          }
          event "添加": Value Change {
            n789 = event-data() -> ("NewVal"=w980:bool)  [unwired: 1 in, 5 out]
            n790 = local read "请输入添加的产品名称"() -> (w977:string)
            n791 = call <vilib>:"Trim Whitespace.vi"("string"=w977) -> ("trimmed string"=w981:string)  [unwired: 1 in]
            n792 = White Space?(1:w981) -> (0:w982:bool)
            n793 = case shown="假" w982 {
              tunnel: w978 -> [w985 _]
              tunnel: w980 -> [w984 _]
              tunnel: w979 -> [w983 _]
              frame False {
                n794 = case shown="真" w984 {
                  tunnel: w985 -> [_ w987]
                  tunnel: w983 -> [_ w986]
                  frame False {
                  }
                  frame True {
                    n795 = for {
                      tunnel: w987 -> [w990] mode=indexing
                      tunnel: w986 -> [w989]
                      n796 = call "Read_Write ParaINI File.vi"("Mode"=enum16{"Read", "Write"}."Write", "Section"="请输入添加的产品名称", "Filepath"=w989, "Ctl Refnum"=w990) -> ()  [unwired: 7 in, 1 out]
                    }
                  }
                }
              }
              frame True {
                w992 = 64 items=["None"=0, "Hand, Error, Stop"=16, "Question"=32, "Exclamation, Warning"=48, "Asterisk, Information"=64] ("icon")
                w993 = 0 items=["OK", "OKCancel", "AbortRetryIgnore", "YesNoCancel", "YesNo", "RetryCancel"] ("buttons")
                n797 = call "信息框（标题、文本、图标）.vi"("icon"=w992, "buttons"=w993, "caption"="添加失败", "text"="请输入产品名称!") -> ()  [unwired: 6 in, 2 out]
              }
            }
          }
          event "产品型号": Value Change {
            n798 = event-data() -> ()  [unwired: 1 in, 6 out]
            n799 = stacked-sequence {
              tunnel: w996 -> [_ w999]
              tunnel: w997 -> [_ w998]
              frame #0 {
              }
              frame #1 {
                n800 = for {
                  tunnel: w999 -> [w1002] mode=indexing
                  tunnel: w998 -> [w1001]
                  n801 = local read "产品型号"() -> (w1000:string)
                  n802 = call "Read_Write ParaINI File.vi"("Mode"=enum16{"Read", "Write"}."Read", "Section"=w1000, "Filepath"=w1001, "Ctl Refnum"=w1002) -> ()  [unwired: 7 in, 1 out]
                }
              }
            }
          }
          event "退出": Value Change {
            n803 = event-data() -> ()  [unwired: 1 in, 6 out]
            n804 = control-ref of="本VI"() -> (w1006:refnum<vi>)
            n805 = invoke class="VI" method="FP.Close"(reference=w1006) -> (reference out=w1004:refnum<vi>, error out=w1005:errorcluster)  [unwired: 2 in, 1 out]
            n806 = Close Reference(reference=w1004, error in (no error)=w1005) -> ()  [unwired: 1 out]
          }
          event "更新": Value Change {
            n807 = event-data() -> ("NewVal"=w1009:bool)  [unwired: 1 in, 5 out]
            n808 = case shown="真" w1009 {
              tunnel: w1008 -> [_ w1012]
              tunnel: w1007 -> [_ w1011]
              frame False {
              }
              frame True {
                n809 = for {
                  tunnel: w1012 -> [w1018]
                  tunnel: w1011 -> [w1017] mode=indexing
                  tunnel: [w1016] -> w1010
                  n810 = local read "产品型号"() -> (w1015:string)
                  n811 = call "Read_Write ParaINI File.vi"("Mode"=enum16{"Read", "Write"}."Write", "Section"=w1015, "Filepath"=w1018, "Ctl Refnum"=w1017) -> ("error out"=w1016:errorcluster)  [unwired: 7 in]
                }
                n812 = case shown="无错误" w1010 {
                  frame No Error {
                    n813 = call "浮动通知.vi"("通知内容"="更新成功！") -> ()  [unwired: 11 in]
                  }
                  frame Error {
                    n814 = call "浮动通知.vi"("通知内容"="更新失败！") -> ()  [unwired: 11 in]
                  }
                }
              }
            }
          }
          event "请输入添加的产品名称": Value Change {
            n815 = event-data() -> ("NewVal"=w1021:string)  [unwired: 1 in, 5 out]
            n816 = control-ref of="产品型号"() -> (w1020:refnum<vi>)
            n817 = property on="属性节点" class="CmbBox"(reference=w1020) -> ("Strings[]"=w1022:string[])  [unwired: 1 in, 2 out]
            n818 = for {
              tunnel: w1021 -> [w1023]
              tunnel: w1022 -> [w1024] mode=indexing
              n819 = Equal?(x=w1023, y=w1024) -> (x = y?=w1025:bool)
              n820 = case shown="真" w1025 {
                tunnel: w1023 -> [_ w1026]
                frame False {
                }
                frame True {
                  n821 = stacked-sequence {
                    tunnel: w1026 -> [w1032 _]
                    frame #0 {
                      w1027 = 64 items=["None"=0, "Hand, Error, Stop"=16, "Question"=32, "Exclamation, Warning"=48, "Asterisk, Information"=64] ("icon")
                      w1028 = 0 items=["OK", "OKCancel", "AbortRetryIgnore", "YesNoCancel", "YesNo", "RetryCancel"] ("buttons")
                      n822 = Concatenate Strings("已经存在产品”" ("text"), w1032, "“\n请勿重复添加！" ("字符串")) -> (w1030:string)
                      n823 = call "信息框（标题、文本、图标）.vi"("icon"=w1027, "buttons"=w1028, "caption"="产品重复", "text"=w1030) -> ()  [unwired: 6 in, 2 out]
                    }
                    frame #1 {
                      n824 = local write "请输入添加的产品名称"("" ("请输入添加的产品名称")) -> ()
                    }
                  }
                }
              }
            }
          }
          event Panel Close? {
            n825 = event-data() -> ()  [unwired: 1 in, 4 out]
            n826 = global write "Global.vi" "程序关闭"(TRUE ("程序关闭")) -> ()
            n827 = control-ref of="本VI"() -> (w1040:refnum<vi>)
            n828 = vi-ref "client.vi"() -> (w1035:refnum<vi>)
            n829 = invoke class="VI" method="FP.Close"(reference=w1040) -> (reference out=w1038:refnum<vi>, error out=w1039:errorcluster)  [unwired: 2 in, 1 out]
            n830 = invoke class="VI" method="FP.Close"(reference=w1035) -> (reference out=w1036:refnum<vi>, error out=w1037:errorcluster)  [unwired: 2 in, 1 out]
            n831 = Close Reference(reference=w1038, error in (no error)=w1039) -> ()  [unwired: 1 out]
            n832 = Close Reference(reference=w1036, error in (no error)=w1037) -> ()  [unwired: 1 out]
            n833 = event-data("Discard?"=TRUE ("放弃？")) -> ()  [unwired: 1 in, 1 out]
          }
          event "进入用户管理": Value Change {
            n834 = event-data() -> ()  [unwired: 1 in, 6 out]
            n835 = vi-ref "User_manager.vi"() -> (w1044:refnum<vi>)
            n836 = call "CallVI.vi"("VI引用"=w1044, "状态"=T1."Maximized") -> ()  [unwired: 11 in, 3 out]
          }
          event "设备故障": Value Change {
            n837 = event-data() -> ()  [unwired: 1 in, 6 out]
            n838 = call "状态改变.vi"("设备状态"=enum16{"设备离线", "设备正常", "设备缺料", "设备故障", "质量报警"}."设备故障") -> ()  [unwired: 11 in]
          }
          event "设备缺料": Value Change {
            n839 = event-data() -> ()  [unwired: 1 in, 6 out]
            n840 = call "状态改变.vi"("设备状态"=enum16{"设备离线", "设备正常", "设备缺料", "设备故障", "质量报警"}."设备缺料") -> ()  [unwired: 11 in]
          }
          event "质量报警": Value Change {
            n841 = event-data() -> ()  [unwired: 1 in, 6 out]
            n842 = call "状态改变.vi"("设备状态"=enum16{"设备离线", "设备正常", "设备缺料", "设备故障", "质量报警"}."质量报警") -> ()  [unwired: 11 in]
          }
        }
        n843 = global read "Global.vi" "程序关闭"() -> (w113:bool)
      }
    }
  }
  n844 = disable-structure shown="禁用" {
    disable-tunnel: _ -> [w1092 _]
    frame Disabled {
      n845 = local read "位移区间2内最小压力(KN)"() -> (w1063:dbl)
      n846 = local read "deviceid"() -> (w1056:string)
      n847 = local read "codeid"() -> (w1058:string)
      n848 = local read "位移区间2内最大压力(KN)"() -> (w1075:dbl)
      n849 = local read "deviceid"() -> (w1068:string)
      n850 = local read "最小压力下限 2"() -> (w1064:dbl)
      n851 = local read "最小压力上限 2"() -> (w1065:dbl)
      n852 = local read "deviceid"() -> (w1130:string)
      n853 = local read "codeid"() -> (w1072:string)
      n854 = local read "codeid"() -> (w1128:string)
      n855 = local read "判定结果2 2"() -> (w1055:string)
      n856 = local read "压装最终位移(mm)"() -> (w1122:dbl)
      n857 = local read "最大压力下限 2"() -> (w1076:dbl)
      n858 = local read "最大压力上限 2"() -> (w1077:dbl)
      n859 = local read "压装最终位移下限"() -> (w1121:dbl)
      n860 = local read "压装最终位移上限"() -> (w1120:dbl)
      n861 = local read "判定结果1 2"() -> (w1074:string)
      n862 = Decimal String To Number(string=w1056, default (0L)=i64 0 ("默认(0 I32)")) -> (number=w1060:i64)  [unwired: 1 in, 1 out]
      n863 = Decimal String To Number(string=w1058, default (0L)=i64 0 ("默认(0 I32)")) -> (number=w1061:i64)  [unwired: 1 in, 1 out]
      n864 = local read "判定结果3"() -> (w1119:string)
      n865 = Decimal String To Number(string=w1068, default (0L)=i64 0 ("默认(0 I32)")) -> (number=w1070:i64)  [unwired: 1 in, 1 out]
      n866 = Decimal String To Number(string=w1072, default (0L)=i64 0 ("默认(0 I32)")) -> (number=w1071:i64)  [unwired: 1 in, 1 out]
      n867 = Decimal String To Number(string=w1130, default (0L)=i64 0 ("默认(0 I32)")) -> (number=w1126:i64)  [unwired: 1 in, 1 out]
      n868 = Decimal String To Number(string=w1128, default (0L)=i64 0 ("默认(0 I32)")) -> (number=w1125:i64)  [unwired: 1 in, 1 out]
      n869 = Bundle(w1060, w1061, "位移区间2内最小压力", "位移区间2内最小压力(KN)"=w1063, "最小压力下限 2"=w1064, "最小压力上限 2"=w1065, "KN", "判定结果2 2"=w1055) -> (w1050:T9)  [unwired: 1 in]
      n870 = Bundle(w1070, w1071, "位移区间2内最大压力", "位移区间2内最大压力(KN)"=w1075, "最大压力下限 2"=w1076, "最大压力上限 2"=w1077, "KN", "判定结果1 2"=w1074) -> (w1051:T10)  [unwired: 1 in]
      n871 = Bundle(w1126, w1125, "压装最终位移", "压装最终位移(mm)"=w1122, "压装最终位移下限"=w1121, "压装最终位移上限"=w1120, "mm", "判定结果3"=w1119) -> (w1081:T11)  [unwired: 1 in]
      n872 = local read "deviceid"() -> (w1118:string)
      n873 = local read "侧铆最大压力(KN)"() -> (w1110:dbl)
      n874 = local read "侧铆最大压力上限"() -> (w1090:dbl)
      n875 = local read "侧铆最大压力下限"() -> (w1091:dbl)
      n876 = local read "codeid"() -> (w1116:string)
      n877 = local read "侧铆判定结果"() -> (w1089:string)
      n878 = local read "位移区间1内最小压力(KN)"() -> (w1133:dbl)
      n879 = local read "deviceid"() -> (w1140:string)
      n880 = local read "codeid"() -> (w1138:string)
      n881 = Decimal String To Number(string=w1118, default (0L)=i64 0 ("默认(0 I32)")) -> (number=w1114:i64)  [unwired: 1 in, 1 out]
      n882 = Decimal String To Number(string=w1116, default (0L)=i64 0 ("默认(0 I32)")) -> (number=w1113:i64)  [unwired: 1 in, 1 out]
      n883 = local read "最小压力下限"() -> (w1132:dbl)
      n884 = local read "最小压力上限"() -> (w1131:dbl)
      n885 = call "GetSQLstring.vi"("联机模式"=w1092) -> ("错误输出"=w1156:errorcluster, "连接字符串"=w1157:string)  [unwired: 9 in]
      n886 = local read "判定结果2"() -> (w1141:string)
      n887 = Decimal String To Number(string=w1140, default (0L)=i64 0 ("默认(0 I32)")) -> (number=w1136:i64)  [unwired: 1 in, 1 out]
      n888 = Decimal String To Number(string=w1138, default (0L)=i64 0 ("默认(0 I32)")) -> (number=w1135:i64)  [unwired: 1 in, 1 out]
      n889 = call-poly <vilib>:"DB Tools Open Connection.vi"("error in (no error)"=w1156, "connection information"=w1157) -> ("error out"=w1158:errorcluster, "connection reference"=w1154:T5)  [unwired: 6 in]
      n890 = Bundle(w1114, w1113, "侧铆最大压力", "侧铆最大压力(KN)"=w1110, "侧铆最大压力下限"=w1091, "侧铆最大压力上限"=w1090, "KN", "侧铆判定结果"=w1089) -> (w1080:T12)  [unwired: 1 in]
      n891 = Bundle(w1136, w1135, "位移区间内最小压力", "位移区间1内最小压力(KN)"=w1133, "最小压力下限"=w1132, "最小压力上限"=w1131, "KN", "判定结果2"=w1141) -> (w1052:T13)  [unwired: 1 in]
      n892 = local read "deviceid"() -> (w1109:string)
      n893 = local read "端铆最大压力0°(KN)"() -> (w1102:dbl)
      n894 = local read "端铆最大压力0°下限"() -> (w1088:dbl)
      n895 = local read "端铆最大压力0°上限"() -> (w1087:dbl)
      n896 = local read "codeid"() -> (w1107:string)
      n897 = local read "端铆判定结果0°"() -> (w1085:string)
      n898 = local read "位移区间1内最大压力(KN)"() -> (w1145:dbl)
      n899 = Decimal String To Number(string=w1109, default (0L)=i64 0 ("默认(0 I32)")) -> (number=w1105:i64)  [unwired: 1 in, 1 out]
      n900 = Decimal String To Number(string=w1107, default (0L)=i64 0 ("默认(0 I32)")) -> (number=w1104:i64)  [unwired: 1 in, 1 out]
      n901 = local read "deviceid"() -> (w1152:string)
      n902 = local read "codeid"() -> (w1148:string)
      n903 = local read "最大压力下限"() -> (w1144:dbl)
      n904 = local read "最大压力上限"() -> (w1143:dbl)
      n905 = local read "判定结果1"() -> (w1146:string)
      n906 = Bundle(w1105, w1104, "端铆最大压力0°", "端铆最大压力0°(KN)"=w1102, "端铆最大压力0°下限"=w1088, "端铆最大压力0°上限"=w1087, "KN", "端铆判定结果0°"=w1085) -> (w1079:T14)  [unwired: 1 in]
      n907 = Decimal String To Number(string=w1152, default (0L)=i64 0 ("默认(0 I32)")) -> (number=w1150:i64)  [unwired: 1 in, 1 out]
      n908 = Decimal String To Number(string=w1148, default (0L)=i64 0 ("默认(0 I32)")) -> (number=w1149:i64)  [unwired: 1 in, 1 out]
      n909 = local read "端铆最大压力45°(KN)"() -> (w1094:dbl)
      n910 = local read "端铆最大压力45°上限"() -> (w1083:dbl)
      n911 = local read "端铆最大压力45°下限"() -> (w1084:dbl)
      n912 = local read "deviceid"() -> (w1101:string)
      n913 = local read "codeid"() -> (w1099:string)
      n914 = local read "端铆判定结果45°"() -> (w1082:string)
      n915 = Bundle(w1150, w1149, "位移区间内最大压力", "位移区间1内最大压力(KN)"=w1145, "最大压力下限"=w1144, "最大压力上限"=w1143, "KN", "判定结果1"=w1146) -> (w1053:T15)  [unwired: 1 in]
      n916 = Decimal String To Number(string=w1101, default (0L)=i64 0 ("默认(0 I32)")) -> (number=w1097:i64)  [unwired: 1 in, 1 out]
      n917 = Decimal String To Number(string=w1099, default (0L)=i64 0 ("默认(0 I32)")) -> (number=w1096:i64)  [unwired: 1 in, 1 out]
      n918 = Bundle(w1097, w1096, "端铆最大压力45°", "端铆最大压力45°(KN)"=w1094, "端铆最大压力45°下限"=w1084, "端铆最大压力45°上限"=w1083, "KN", "端铆判定结果45°"=w1082) -> (w1078:T16)  [unwired: 1 in]
      n919 = Build Array(w1053, w1052, w1051, w1050, w1081, w1080, w1079, w1078) -> (w1048:T17)
      n920 = for {
        tunnel: w1048 -> [w1159] mode=indexing
        tunnel: w1154 -> [w1162]
        shift-right: [w1160] -> w1049
        shift-left: w1158 -> [w1166]
        w1163 = string[] ["DEVICE_ID", "CODE_ID", "TEST_NAME", "TEST_VALUE", "TEST_VALUE_MIN", "TEST_VALUE_MAX", "TEST_VALUE_UNIT", "TEST_VALUE_RESULT"] ("columns")
        w1164 = "Test" ("table")
        n921 = call <vilib>:"DB Tools Insert Data.vi"("data"=w1159, "error in (no error)"=w1166, "columns"=w1163, "table"=w1164, "connection reference"=w1162) -> ("error out"=w1165:errorcluster, "connection reference out"=w1161:T5)  [unwired: 5 in]
        n922 = case shown="错误" w1165 {
          selector: w1165 -> [w1167 w1192]
          tunnel: w1163 -> [_ w1189]
          tunnel: w1161 -> [w1168 w1174]
          tunnel: w1164 -> [_ w1193]
          tunnel: w1159 -> [_ w1183]
          tunnel: [w1168 w1173] -> _
          tunnel: [w1167 w1172] -> w1160
          frame No Error {
          }
          frame Error {
            n923 = Delete From Array(array=w1189, length=1 ("长度"), index=2 ("索引")) -> (array with subset deleted=w1190:string[])  [unwired: 1 out]
            n924 = call <vilib>:"Clear Errors.vi"("error in (no error)"=w1192) -> ("error out"=w1191:errorcluster)  [unwired: 5 in, 1 out]
            n925 = Unbundle(w1183) -> (w1182:i64, w1170:i64, w1175:string, "端铆最大压力45°(KN)"=w1181:dbl, "端铆最大压力45°下限"=w1180:dbl, "端铆最大压力45°上限"=w1179:dbl, w1178:string, "端铆判定结果45°"=w1177:string)
            n926 = Bundle(w1182, w1170, "端铆最大压力45°(KN)"=w1181, "端铆最大压力45°下限"=w1180, "端铆最大压力45°上限"=w1179, w1178, "端铆判定结果45°"=w1177) -> (w1176:T18)  [unwired: 1 in]
            n927 = Number To Decimal String(number=w1170) -> (decimal integer string=w1169:string)  [unwired: 1 in]
            n928 = Concatenate Strings("WHERE TEST_NAME ='" ("condition"), w1175, "'", "AND CODE_ID =" ("condition"), w1169) -> (w1185:string)
            n929 = call <vilib>:"DB Tools Update Data.vi"("condition"=w1185, "data"=w1176, "error in (no error)"=w1191, "columns"=w1190, "table"=w1193, "connection reference"=w1174) -> ("error out"=w1172:errorcluster, "connection reference out"=w1173:T5)  [unwired: 4 in]
          }
        }
      }
      n930 = call <vilib>:"Simple Error Handler.vi"("error in (no error)"=w1049) -> ()  [unwired: 4 in, 5 out]
      n931 = call <vilib>:"Simple Error Handler.vi"("error in (no error)"=w1049) -> ()  [unwired: 4 in, 5 out]
    }
    frame Enabled {
    }
  }
